vi "Main.vi"() -> ()   [LabVIEW 2020]
doc: "Use this template to build a simple state machine design pattern. Each state executes code and determines which state to transition to."
uses:
  controls/State.ctl
  controls/Data.ctl
  <vilib>/Utility/file.llb/Write Delimited Spreadsheet (string).vi
panel:
  in  "Operator":string(combo)
  in  "Run Lift-Off Pulses":bool
  out "Number of layers":i32
  out "Build":string
  in  "Refresh Supplies":bool
  out "Current now [A]":dbl format="%#.2f"
  in  "Wafer Box":string(combo)="(i)(1)"
  out "Elapsed Time [s]":dbl min=0.0 step=1.0 format="%#.1f"
  in  "Run Lift-Off Pulses\nAfter Etching":bool=TRUE
  in  "Edit Lift-Off Pulses":bool
  in  "Start Etching":bool
  in  "Everyting Correct":bool
  in  "Total Etch Time [s]":u32=2400 step=1
  in  "Wait Time [ms]":u32=2 step=1
  in  "Pulse 2 Time [ms]":u32=2 step=1
  in  "Pulse 1 Time [ms]":u32=2 step=1
  out "[A]":dbl=50.0 min=0.0 max=500.0 step=0.1 format="%#.2g"
  in  "Pulse 2 [mA/cm²]":dbl=50.0 min=0.0 max=900.0 step=0.1 format="%#.3g"
  out "[A]":dbl=50.0 min=0.0 max=500.0 step=0.1 format="%#.2g"
  in  "Pulse 1 [mA/cm²]":dbl=50.0 min=0.0 max=900.0 step=0.1 format="%#.3g"
  out "XY Graph":cluster{"X":dbl[], "Y":dbl[]}[](graph)
  in  "Etch type":T1(tab)
  in  "Current density (mA/cm²)":dbl=30.0 format="%#.2g"
  in  "Current density 1 [mA/cm²]":dbl=50.0 min=0.0 max=500.0 step=0.1 format="%#.2g"
  in  "Current density 2 [mA/cm²]":dbl=200.0 min=0.0 max=500.0 step=0.1 format="%#.2g"
  in  "Pulse time 1 [ms]":u32=2200 step=1
  in  "Pulse time 2 [ms]":u32=350 step=1
  in  "Stop time [ms]":u32=1000 step=1
  in  "Start Current Time [ms]":u32=2000 step=1
  in  "Start Current density [mA/cm²]":dbl=30.0 min=0.0 max=500.0 step=0.1 format="%#.2g"
  in  "Power order":dbl=1.0 min=0.0 step=0.1 format="%#.1g"
  in  "Increment time span [ms]":u32=250 step=1
  in  "Current Density Increment [mA/cm²/s^(power order)]":dbl=1.0 min=0.0 max=500.0 step=0.1 format="%#.6g"
  in  "Etch Surface Area [cm²]":dbl min=0.0 max=1000.0 step=0.1 format="%#.2f"
  in  "Etch Cell":i32(slide) scale=0.0..3.0
  in  "Power Supply":u16(ring)
  in  "Exit":bool
  # "University of Eastern Finland\nJoakim Riikonen / Konstantin Tamarov"
  # "The Ultimate PSi Etching Software"
  # "Etch Cell and Etch Surface Area"
  # "Etch Program"
  # "Lift-Off Pulses"
  # "Start Etching"
  # "Start with short period of contant current to initiate pores"
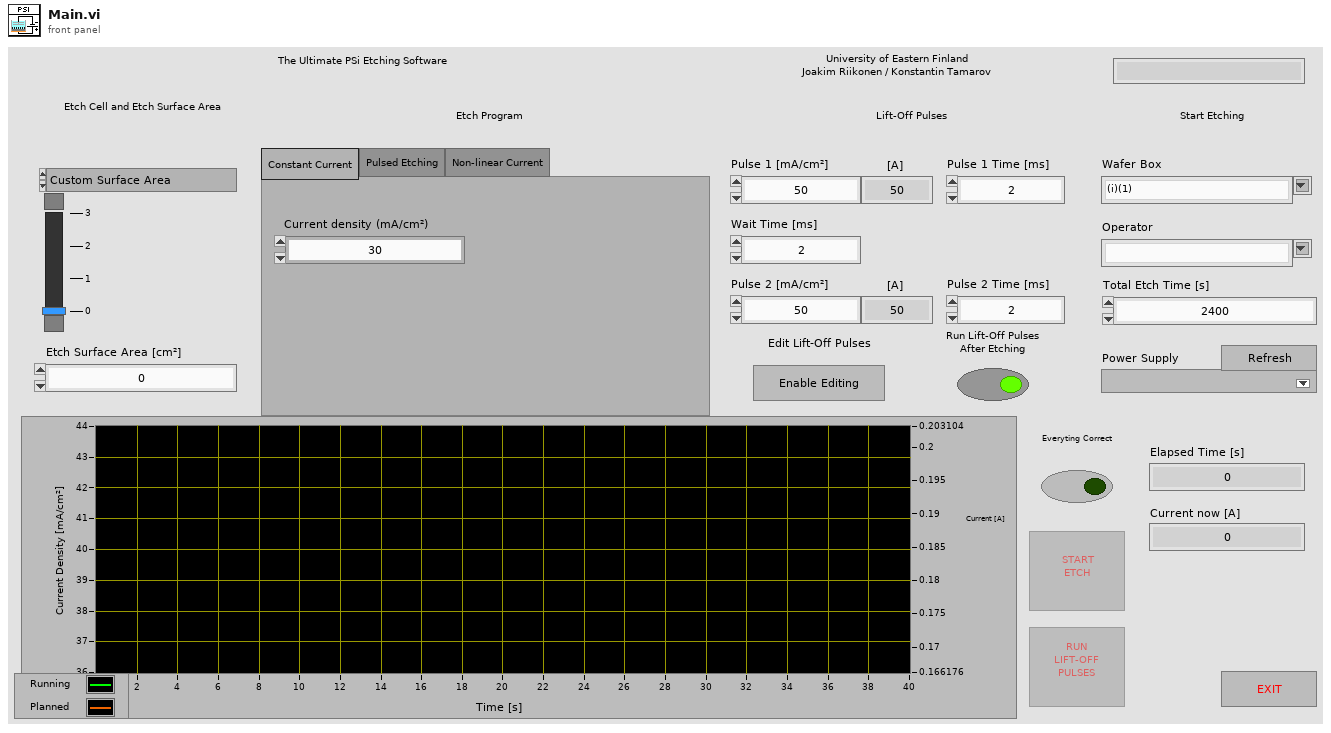
[diagram p1: front panel]
types:
  T1 = enum32{"Constant Current", "Pulsed Etching", "Non-linear Current"}
  T2 = typedef "State.ctl" = enum16{"Initialize", "Wait for Message", "Etch Cell Changed", "LiftOff Pulse Changed", "Enable Editing Pulses Clicked", "Etch Type Changed", "Refresh Supplies Clicked", "Etch Parameters Changed", "Prepare Etch Program", "Check Power Supplies", "Check Max Current", "Prepare Graph", "Before Etch", "Prepare Log", "Etch Running", "Stop Etch Clicked", "LiftOff Pulses", "After Etch", "Exit"}
  T3 = typedef "Data.ctl" = cluster{"Power Supplies":cluster{"Full Name":string[], "Supply Model":string[], "Supply Address":string[], "Max Voltage (V)":dbl[], "Max Current (A)":dbl[]}, "Etch Cell Data":cluster{"Cell Type":string[], "Power Supply Model":string[], "Etch Surface Area (cm2)":dbl[], "LiftOff Pulse 1 (mA/cm2)":dbl[], "LiftOff Time 1 (ms)":u32[], "LiftOff Wait Time 1 (ms)":u32[], "LiftOff Pulse 2 (mA/cm2)":dbl[], "LiftOff Time 2 (ms)":i32[]}, "Etch Program":cluster{"Current Time [ms]":u32[], "Current Density [mA/cm2]":dbl[], "Current [A]":dbl[]}, "Graph Data":cluster{"X":dbl[], "Y":dbl[]}, "Selected VISA":string, "Selected Voltage Limit":dbl, "Log":string[], "Etch Result":string, "Etch Finished Correctly":bool, "Only LiftOff Pulses":bool}
  T4 = enum8{"Enabled", "Disabled", "Disabled and Grayed Out"}
  T5 = cluster{"Current Density [mA/cm2]":dbl[], "Current [A]":dbl[], "Current Time [ms]":u32[]}
  T6 = cluster{"array":string[], "array":string[], "array":string[], "array":dbl[], "array":dbl[]}
  T7 = cluster{"array":string[], "array":string[], "array":dbl[], "array":dbl[], "array":u32[], "array":u32[], "array":dbl[], "array":i32[]}
  T8 = cluster{"array":i32[], "array":dbl[], "array":dbl[]}
  T9 = cluster{"Current Time [ms]":u32[], "Current Density [mA/cm2]":dbl[], "Current [A]":dbl[]}
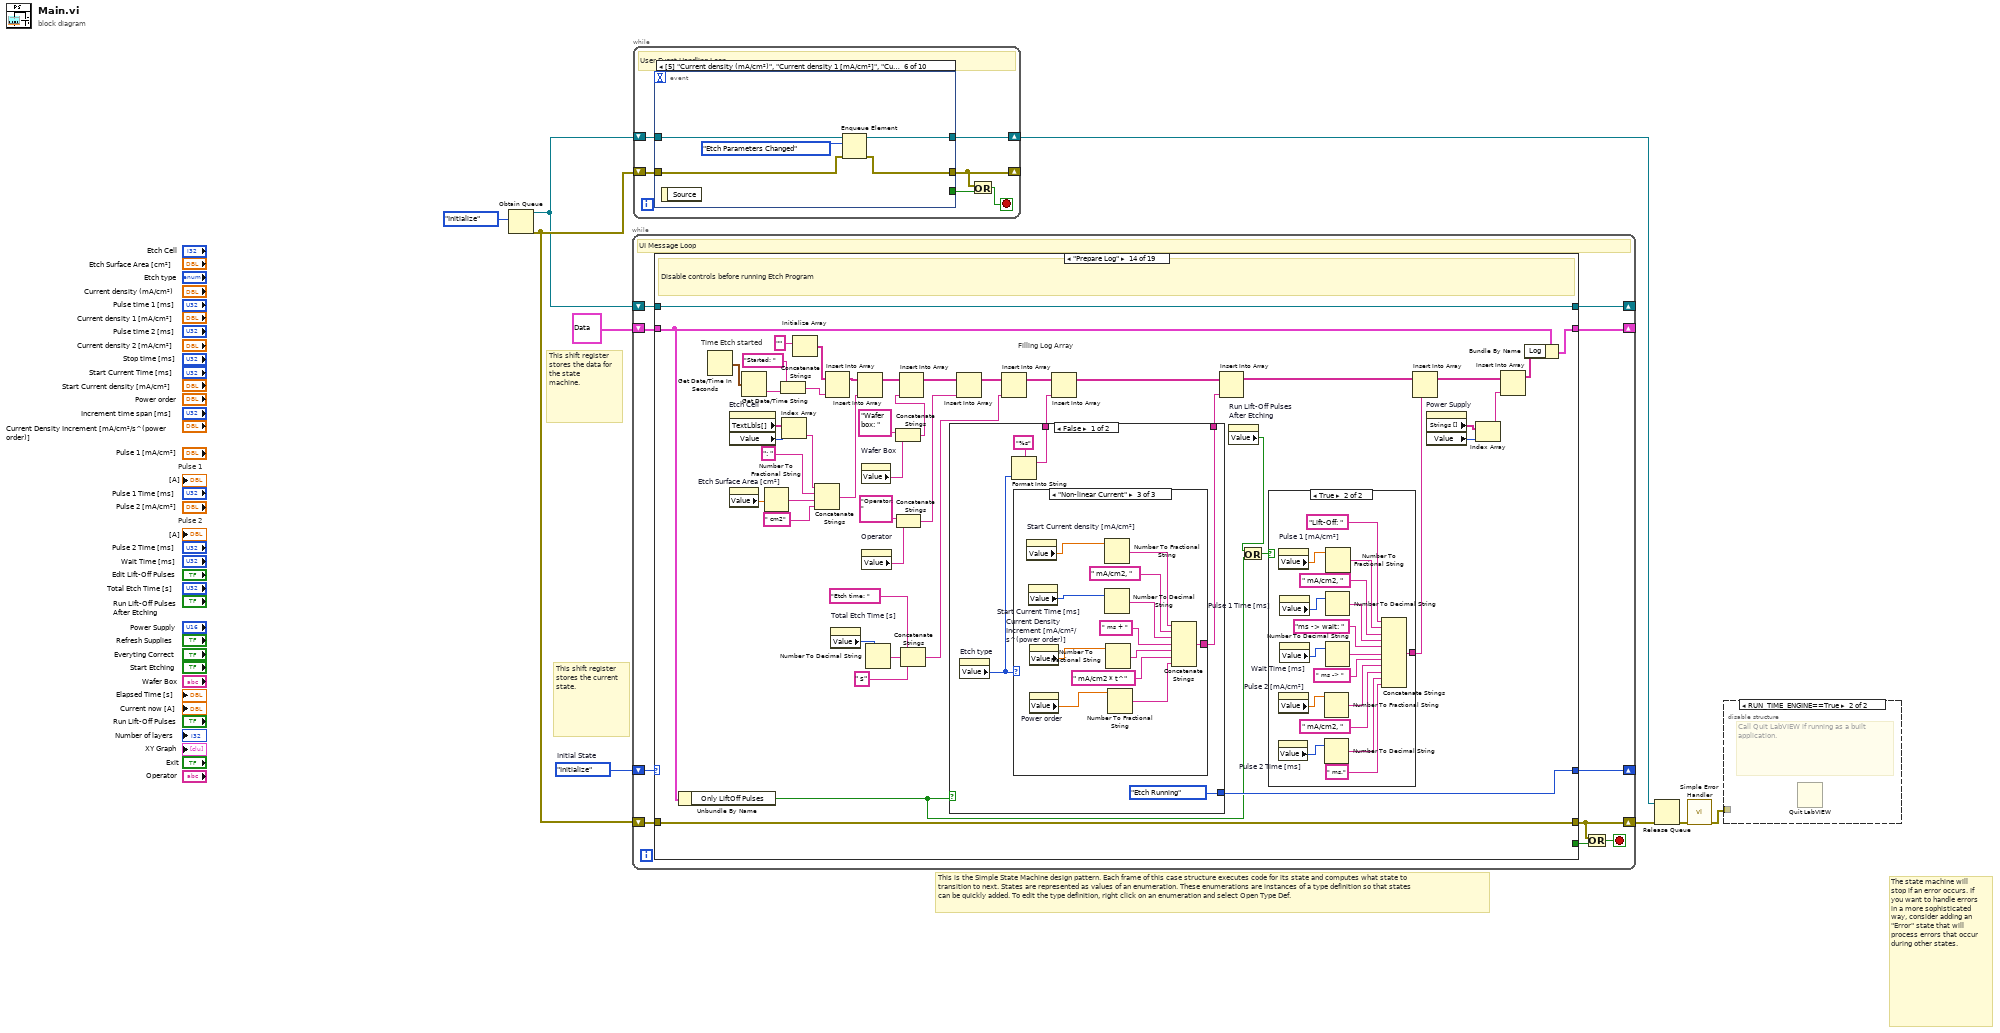
[diagram p0: block diagram]
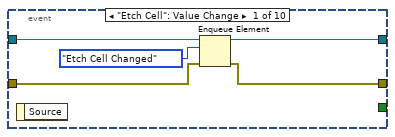
[diagram p2: hidden frame]
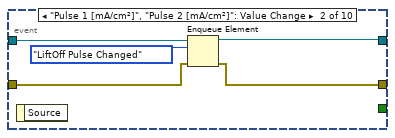
[diagram p3: hidden frame]
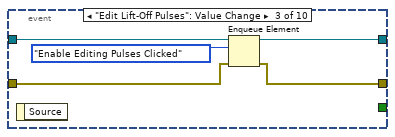
[diagram p4: hidden frame]
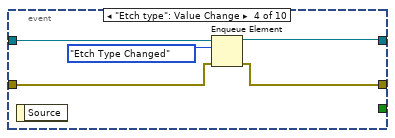
[diagram p5: hidden frame]
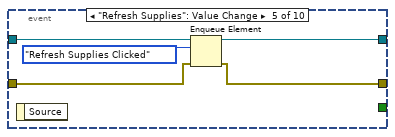
[diagram p6: hidden frame]
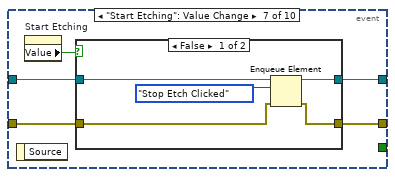
[diagram p7: hidden frame]
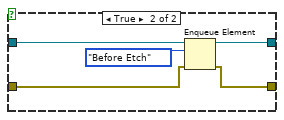
[diagram p8: hidden frame]
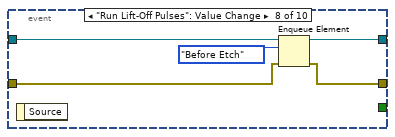
[diagram p9: hidden frame]
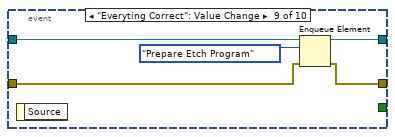
[diagram p10: hidden frame]
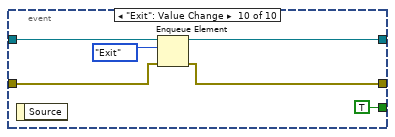
[diagram p11: hidden frame]
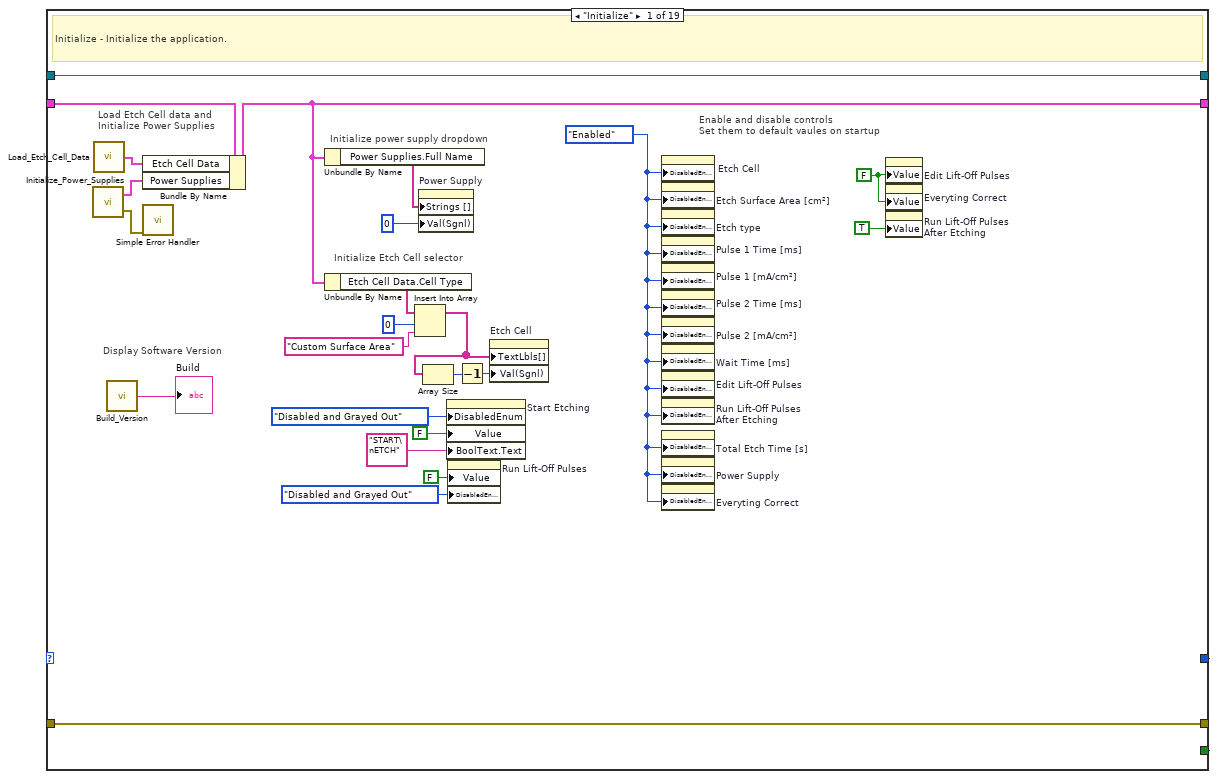
[diagram p13: hidden frame]
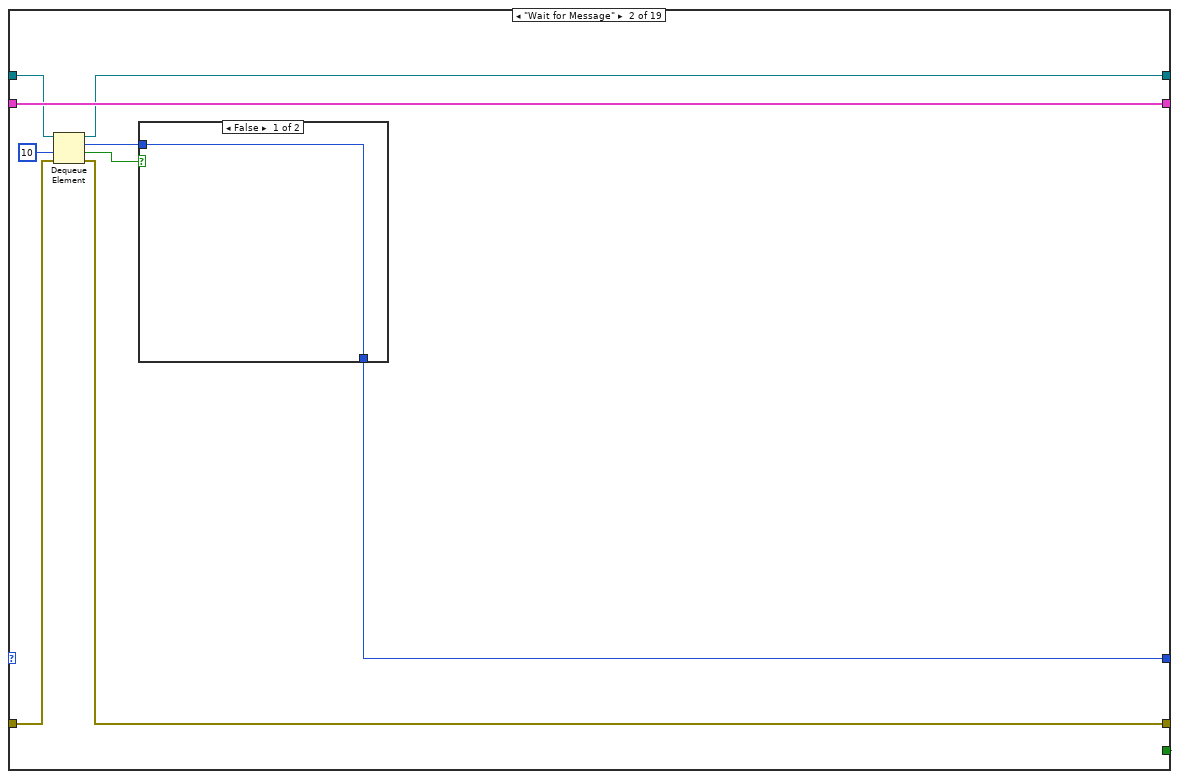
[diagram p14: hidden frame]
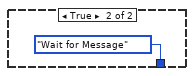
[diagram p15: hidden frame]
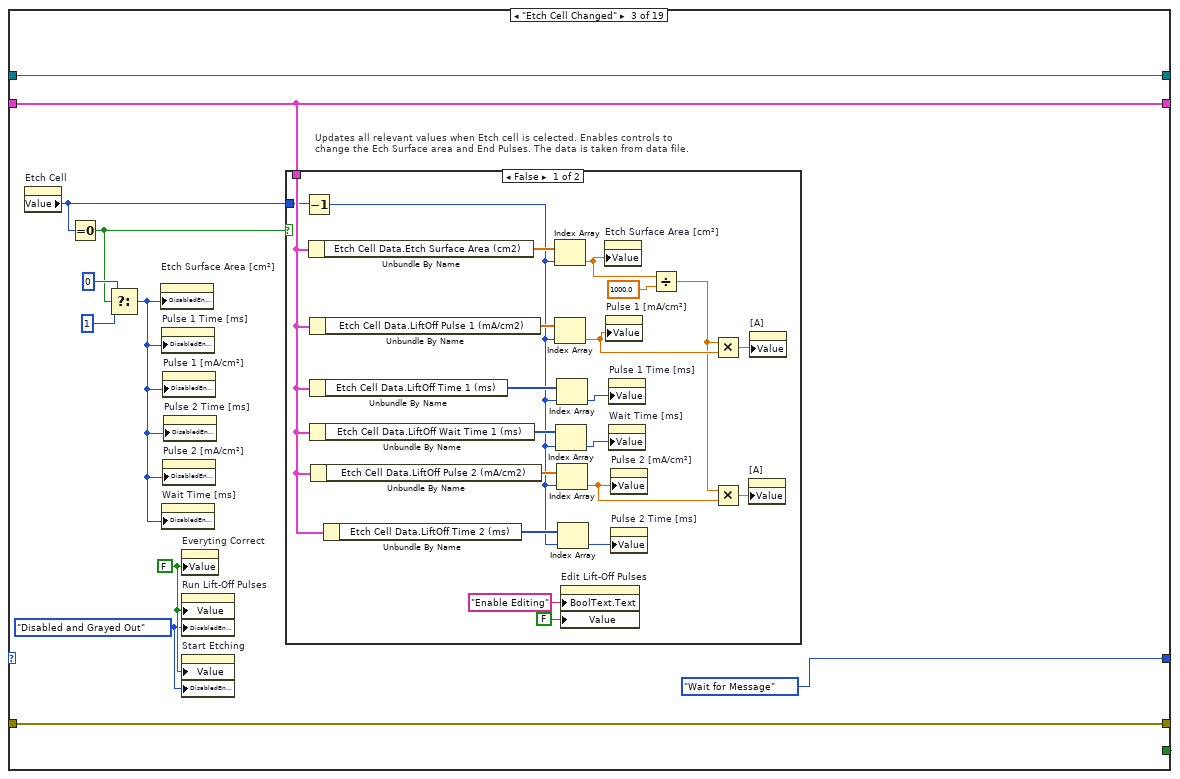
[diagram p16: hidden frame]
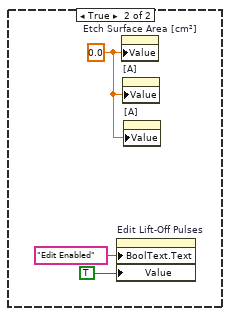
[diagram p17: hidden frame]
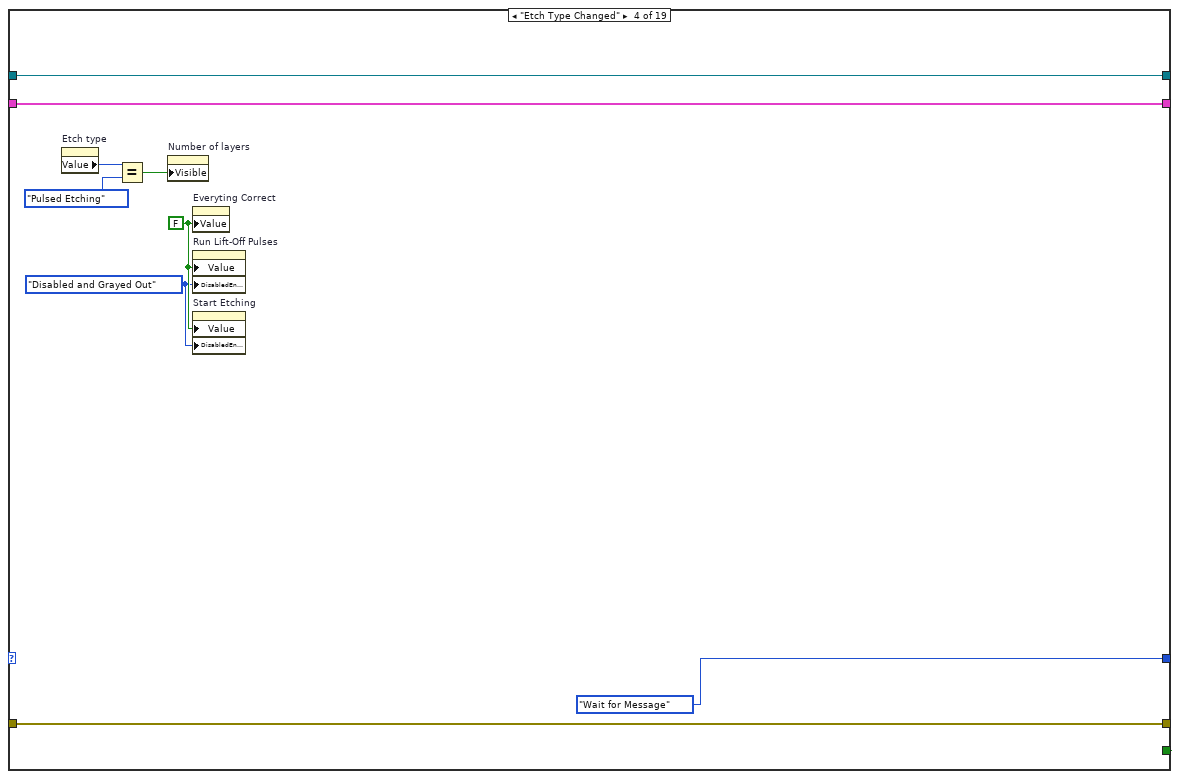
[diagram p18: hidden frame]
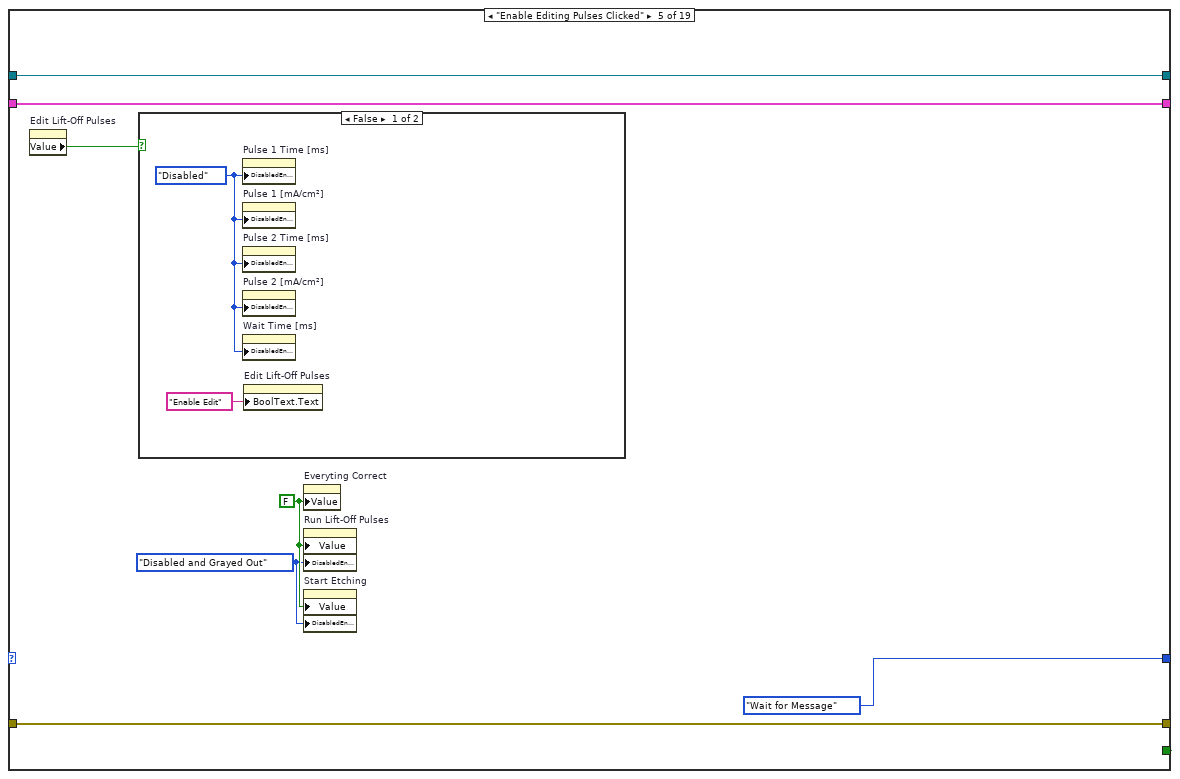
[diagram p19: hidden frame]
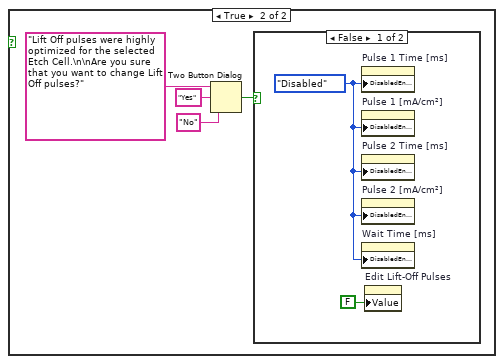
[diagram p20: hidden frame]
diagram:
  w5 = State."Initialize"  # Initial State
  # "Pulse 2"
  # "Pulse 1"
  # "The state machine will stop if an error occurs. If you want to handle errors in a more sophisticated way, consider adding an \"Error\" state that will process errors that occur during other states."
  # "This shift register stores the data for the state machine."
  # "This is the Simple State Machine design pattern. Each frame of this case structure executes code for its state and computes what state to transition to next. States are represented as values of an enumeration. These enumerations are instances of a type definition so that states can be quickly added. To edit the type definition, right click on an enumeration and select Open Type Def."
  # "This shift register stores the current state."
  n1 = Obtain Queue(element data type=State."Initialize" ("element")) -> (queue out=w3:refnum<queue>, error out=w7:errorcluster)  [unwired: 4 in, 1 out]
  n2 = while {
    shift-right: [w19] -> _
    shift-left: w5 -> [w12]
    shift-right: [w13] -> _
    shift-left: T3 {"Power Supplies"={"Full Name"=[], "Supply Model"=[], "Supply Address"=[], "Max Voltage (V)"=[], "Max Current (A)"=[]}, "Etch Cell Data"={"Cell Type"=[], "Power Supply Model"=[], "Etch Surface Area (cm2)"=[], "LiftOff Pulse 1 (mA/cm2)"=[], "LiftOff Time 1 (ms)"=[], "LiftOff Wait Time 1 (ms)"=[], "LiftOff Pulse 2 (mA/cm2)"=[], "LiftOff Time 2 (ms)"=[]}, "Etch Program"={"Current Time [ms]"=[], "Current Density [mA/cm2]"=[], "Current [A]"=[]}, "Graph Data"={"X"=[], "Y"=[]}, "Selected VISA"="", "Selected Voltage Limit"=0.0, "Log"=[], "Etch Result"="", "Etch Finished Correctly"=FALSE, "Only LiftOff Pulses"=FALSE} ("Data") -> [w14]
    shift-right: [w15] -> w2
    shift-left: w7 -> [w18]
    shift-right: [w10] -> _
    shift-left: w3 -> [w11]
    stop <- w16 stop-if-true
    # "UI Message Loop"
    n3 = case shown="\"Prepare Log\"" w12 {
      tunnel: [w45 w46 State."Wait for Message" ("(Value Not Used)") State."Wait for Message" ("(Value Not Used)") State."Wait for Message" ("(Value Not Used)") State."Wait for Message" ("(Value Not Used)") State."Wait for Message" ("(Value Not Used)") State."Wait for Message" ("(Value Not Used)") w156 w288 w325 w384 State."Prepare Log" ("Next State") w437 w591 State."After Etch" ("next state") w703 w746 State."LiftOff Pulses" ("(Value Not Used)")] -> w19
      tunnel: [w44 FALSE ("Stop Loop?") FALSE ("Stop Loop?") FALSE ("Stop Loop?") FALSE ("Stop Loop?") FALSE ("Stop Loop?") FALSE ("Stop Loop?") FALSE ("Stop Loop?") w161 FALSE ("Stop Loop?") FALSE ("Stop Loop?") FALSE ("Stop Loop?") w424 w439 w590 FALSE ("Stop Loop?") w706 w744 FALSE ("Stop Loop?")] -> w17
      tunnel: w14 -> [w43 w55 w63 w103 w111 w135 w141 w154 w158 w292 w328 w365 w413 w438 w557 w648 w705 w745 w751]
      tunnel: [w24 w55 w63 w103 w111 w135 w140 w154 w157 w292 w328 w364 w416 w458 w576 w648 w705 w745 w751] -> w13
      tunnel: w18 -> [w26 w52 w69 w102 w110 w134 w137 w153 w160 w296 w331 w391 w422 w443 w538 w653 w707 w743 w750]
      tunnel: [w26 w51 w69 w102 w110 w134 w137 w153 w160 w296 w331 w391 w422 w443 w537 w653 w707 w743 w750] -> w15
      tunnel: w11 -> [w22 w54 w62 w97 w109 w133 w147 w152 w155 w287 w314 w346 w420 w440 w545 w647 w704 w742 w749]
      tunnel: [w22 w53 w62 w97 w109 w133 w147 w152 w155 w287 w314 w346 w420 w440 w544 w647 w704 w742 w749] -> w10
      frame "Initialize" {
        w31 = T4."Enabled" ("Disabled")
        w37 = FALSE ("Edit Lift-Off Pulses")
        w44 = FALSE  # Stop Loop?
        w45 = State."Wait for Message"  # Next State
        # "Initialize Etch Cell selector"
        # "Enable and disable controls\nSet them to default vaules on startup"
        # "Initialize power supply dropdown"
        # "Display Software Version"
        # "Load Etch Cell data and\nInitialize Power Supplies"
        # "Initialize - Initialize the application."
        n4 = call "Initialize_Power_Supplies.vi"() -> ("error out"=w20:errorcluster, "Available Power Supplies"=w21:T6)  [unwired: 2 in]
        n5 = call "Load_Etch_Cell_Data.vi"() -> ("Etch Cell Data"=w38:T7)  [unwired: 1 in]
        n6 = call "Build_Version.vi"() -> ("Version"=→"Build":string)  [unwired: 1 in]
        n7 = Bundle By Name(cluster=w43, "Etch Cell Data"=w38, "Power Supplies"=w21) -> (w24:T3)
        n8 = call <vilib>:"Simple Error Handler.vi"("error in (no error)"=w20) -> ()  [unwired: 4 in, 5 out]
        n9 = Unbundle By Name(w24) -> ("Power Supplies.Full Name"=w25:string[])
        n10 = Unbundle By Name(w24) -> ("Etch Cell Data.Cell Type"=w42:string[])
        n11 = Insert Into Array(array=w42, index=0, new element="Custom Surface Area" ("new element/subarray")) -> (w39:string[])
        n12 = property on="Power Supply" class="Ring (strict)"("Strings []"=w25, "Val(Sgnl)"=u16 0 ("Value (Signaling)")) -> ()  [unwired: 2 in, 2 out]
        n13 = Array Size(array=w39) -> (size(s)=w33:i32)
        n14 = property on="Start Etching" class="Bool (strict)"("DisabledEnum"=T4."Disabled and Grayed Out" ("Disabled"), "Value"=FALSE ("Start Etching"), "BoolText.Text"="START\nETCH" ("Boolean Text.Text")) -> ()  [unwired: 2 in, 2 out]
        n15 = property on="Run Lift-Off Pulses" class="Bool (strict)"("Value"=FALSE ("Run Lift-Off Pulses"), "DisabledEnum"=T4."Disabled and Grayed Out" ("Disabled")) -> ()  [unwired: 2 in, 2 out]
        n16 = Decrement(x=w33) -> (x-1=w23:i32)
        n17 = property on="Etch Cell" class="Slide (strict)"("TextLbls[]"=w39, "Val(Sgnl)"=w23) -> ()  [unwired: 2 in, 2 out]
        n18 = property on="Etch Cell" class="Slide (strict)"("DisabledEnum"=w31) -> ()  [unwired: 2 in, 2 out]
        n19 = property on="Etch Surface Area [cm²]" class="DigNum (strict)"("DisabledEnum"=w31) -> ()  [unwired: 2 in, 2 out]
        n20 = property on="Etch type" class="TabCtl (strict)"("DisabledEnum"=w31) -> ()  [unwired: 2 in, 2 out]
        n21 = property on="Pulse 1 Time [ms]" class="DigNum (strict)"("DisabledEnum"=w31) -> ()  [unwired: 2 in, 2 out]
        n22 = property on="Pulse 1 [mA/cm²]" class="DigNum (strict)"("DisabledEnum"=w31) -> ()  [unwired: 2 in, 2 out]
        n23 = property on="Pulse 2 Time [ms]" class="DigNum (strict)"("DisabledEnum"=w31) -> ()  [unwired: 2 in, 2 out]
        n24 = property on="Pulse 2 [mA/cm²]" class="DigNum (strict)"("DisabledEnum"=w31) -> ()  [unwired: 2 in, 2 out]
        n25 = property on="Wait Time [ms]" class="DigNum (strict)"("DisabledEnum"=w31) -> ()  [unwired: 2 in, 2 out]
        n26 = property on="Edit Lift-Off Pulses" class="Bool (strict)"("DisabledEnum"=w31) -> ()  [unwired: 2 in, 2 out]
        n27 = property on="Run Lift-Off Pulses\nAfter Etching" class="Bool (strict)"("DisabledEnum"=w31) -> ()  [unwired: 2 in, 2 out]
        n28 = property on="Total Etch Time [s]" class="DigNum (strict)"("DisabledEnum"=w31) -> ()  [unwired: 2 in, 2 out]
        n29 = property on="Power Supply" class="Ring (strict)"("DisabledEnum"=w31) -> ()  [unwired: 2 in, 2 out]
        n30 = property on="Everyting Correct" class="Bool (strict)"("DisabledEnum"=w31) -> ()  [unwired: 2 in, 2 out]
        n31 = property on="Edit Lift-Off Pulses" class="Bool (strict)"("Value"=w37) -> ()  [unwired: 2 in, 2 out]
        n32 = property on="Everyting Correct" class="Bool (strict)"("Value"=w37) -> ()  [unwired: 2 in, 2 out]
        n33 = property on="Run Lift-Off Pulses\nAfter Etching" class="Bool (strict)"("Value"=TRUE ("Run Lift-Off Pulses\nAfter Etching")) -> ()  [unwired: 2 in, 2 out]
      }
      frame "Wait for Message" {
        n34 = Dequeue Element(queue=w54, timeout in ms (-1)=10, error in (no error)=w52) -> (queue out=w53:refnum<queue>, element=w47:T2, timed out?=w48:bool, error out=w51:errorcluster)
        n35 = case shown="False" w48 {
          tunnel: w47 -> [w56 _]
          tunnel: [w56 State."Wait for Message" ("(Value Not Used)")] -> w46
          frame False {
          }
          frame True {
          }
        }
      }
      frame "Etch Cell Changed" {
        w58 = T4."Disabled and Grayed Out" ("Disabled")
        w59 = FALSE ("Everyting Correct")
        # "Updates all relevant values when Etch cell is celected. Enables controls to\nchange the Ech Surface area and End Pulses. The data is taken from data file."
        n36 = property on="Etch Cell" class="Slide (strict)"() -> ("Value"=w64:i32)  [unwired: 2 in, 2 out]
        n37 = Equal To 0?(x=w64) -> (x = 0?=w65:bool)
        n38 = Select(t=i8 0, s=w65, f=i8 1) -> (s? t:f=w68:i8)
        n39 = property on="Etch Surface Area [cm²]" class="DigNum (strict)"("DisabledEnum"=w68) -> ()  [unwired: 2 in, 2 out]
        n40 = property on="Pulse 1 Time [ms]" class="DigNum (strict)"("DisabledEnum"=w68) -> ()  [unwired: 2 in, 2 out]
        n41 = property on="Wait Time [ms]" class="DigNum (strict)"("DisabledEnum"=w68) -> ()  [unwired: 2 in, 2 out]
        n42 = property on="Pulse 1 [mA/cm²]" class="DigNum (strict)"("DisabledEnum"=w68) -> ()  [unwired: 2 in, 2 out]
        n43 = property on="Pulse 2 [mA/cm²]" class="DigNum (strict)"("DisabledEnum"=w68) -> ()  [unwired: 2 in, 2 out]
        n44 = property on="Pulse 2 Time [ms]" class="DigNum (strict)"("DisabledEnum"=w68) -> ()  [unwired: 2 in, 2 out]
        n45 = property on="Everyting Correct" class="Bool (strict)"("Value"=w59) -> ()  [unwired: 2 in, 2 out]
        n46 = property on="Run Lift-Off Pulses" class="Bool (strict)"("Value"=w59, "DisabledEnum"=w58) -> ()  [unwired: 2 in, 2 out]
        n47 = property on="Start Etching" class="Bool (strict)"("Value"=w59, "DisabledEnum"=w58) -> ()  [unwired: 2 in, 2 out]
        n48 = case shown="False" w65 {
          tunnel: w64 -> [w73 _]
          tunnel: w63 -> [w86 _]
          frame False {
            n49 = Decrement(x=w73) -> (x-1=w72:i32)
            n50 = Unbundle By Name(w86) -> ("Etch Cell Data.Etch Surface Area (cm2)"=w90:dbl[])
            n51 = Unbundle By Name(w86) -> ("Etch Cell Data.LiftOff Pulse 1 (mA/cm2)"=w89:dbl[])
            n52 = Unbundle By Name(w86) -> ("Etch Cell Data.LiftOff Time 1 (ms)"=w88:u32[])
            n53 = Unbundle By Name(w86) -> ("Etch Cell Data.LiftOff Wait Time 1 (ms)"=w85:u32[])
            n54 = Unbundle By Name(w86) -> ("Etch Cell Data.LiftOff Pulse 2 (mA/cm2)"=w84:dbl[])
            n55 = Unbundle By Name(w86) -> ("Etch Cell Data.LiftOff Time 2 (ms)"=w83:i32[])
            n56 = Index Array(array=w90, index=w72) -> (element=w78:dbl)
            n57 = Index Array(array=w89, index=w72) -> (element=w80:dbl)
            n58 = Index Array(array=w85, index=w72) -> (element=w82:u32)
            n59 = Index Array(array=w88, index=w72) -> (element=w87:u32)
            n60 = Index Array(array=w84, index=w72) -> (element=w79:dbl)
            n61 = Index Array(array=w83, index=w72) -> (element=w81:i32)
            n62 = property on="Edit Lift-Off Pulses" class="Bool (strict)"("BoolText.Text"="Enable Editing" ("Boolean Text.Text"), "Value"=FALSE ("Edit Lift-Off Pulses")) -> ()  [unwired: 2 in, 2 out]
            n63 = property on="Etch Surface Area [cm²]" class="DigNum (strict)"("Value"=w78) -> ()  [unwired: 2 in, 2 out]
            n64 = property on="Pulse 1 [mA/cm²]" class="DigNum (strict)"("Value"=w80) -> ()  [unwired: 2 in, 2 out]
            n65 = property on="Pulse 1 Time [ms]" class="DigNum (strict)"("Value"=w87) -> ()  [unwired: 2 in, 2 out]
            n66 = property on="Wait Time [ms]" class="DigNum (strict)"("Value"=w82) -> ()  [unwired: 2 in, 2 out]
            n67 = property on="Pulse 2 [mA/cm²]" class="DigNum (strict)"("Value"=w79) -> ()  [unwired: 2 in, 2 out]
            n68 = property on="Pulse 2 Time [ms]" class="DigNum (strict)"("Value"=w81) -> ()  [unwired: 2 in, 2 out]
            n69 = Divide(x=w78, y=1000.0) -> (x/y=w77:dbl)
            n70 = Multiply(x=w77, y=w80) -> (x*y=w71:dbl)
            n71 = Multiply(x=w77, y=w79) -> (x*y=w70:dbl)
            n72 = property on="[A]" class="DigNum (strict)"("Value"=w70) -> ()  [unwired: 2 in, 2 out]
            n73 = property on="[A]" class="DigNum (strict)"("Value"=w71) -> ()  [unwired: 2 in, 2 out]
          }
          frame True {
            w91 = 0.0 ("Etch Surface Area (cm²)")
            n74 = property on="Edit Lift-Off Pulses" class="Bool (strict)"("BoolText.Text"="Edit Enabled" ("Boolean Text.Text"), "Value"=TRUE ("Edit Lift-Off Pulses")) -> ()  [unwired: 2 in, 2 out]
            n75 = property on="Etch Surface Area [cm²]" class="DigNum (strict)"("Value"=w91) -> ()  [unwired: 2 in, 2 out]
            n76 = property on="[A]" class="DigNum (strict)"("Value"=w91) -> ()  [unwired: 2 in, 2 out]
            n77 = property on="[A]" class="DigNum (strict)"("Value"=w91) -> ()  [unwired: 2 in, 2 out]
          }
        }
      }
      frame "Etch Type Changed" {
        w100 = T4."Disabled and Grayed Out" ("Disabled")
        w101 = FALSE ("Everyting Correct")
        n78 = property on="Etch type" class="TabCtl (strict)"() -> ("Value"=w96:T1)  [unwired: 2 in, 2 out]
        n79 = Equal?(x=w96, y=T1."Pulsed Etching") -> (x = y?=w94:bool)
        n80 = property on="Number of layers" class="DigNum (strict)"("Visible"=w94) -> ()  [unwired: 2 in, 2 out]
        n81 = property on="Everyting Correct" class="Bool (strict)"("Value"=w101) -> ()  [unwired: 2 in, 2 out]
        n82 = property on="Run Lift-Off Pulses" class="Bool (strict)"("Value"=w101, "DisabledEnum"=w100) -> ()  [unwired: 2 in, 2 out]
        n83 = property on="Start Etching" class="Bool (strict)"("Value"=w101, "DisabledEnum"=w100) -> ()  [unwired: 2 in, 2 out]
      }
      frame "Enable Editing Pulses Clicked" {
        w105 = T4."Disabled and Grayed Out" ("Disabled")
        w106 = FALSE ("Everyting Correct")
        n84 = property on="Edit Lift-Off Pulses" class="Bool (strict)"() -> ("Value"=w104:bool)  [unwired: 2 in, 2 out]
        n85 = case shown="False" w104 {
          frame False {
            w112 = T4."Disabled" ("Disabled")
            n86 = property on="Pulse 1 Time [ms]" class="DigNum (strict)"("DisabledEnum"=w112) -> ()  [unwired: 2 in, 2 out]
            n87 = property on="Pulse 1 [mA/cm²]" class="DigNum (strict)"("DisabledEnum"=w112) -> ()  [unwired: 2 in, 2 out]
            n88 = property on="Pulse 2 Time [ms]" class="DigNum (strict)"("DisabledEnum"=w112) -> ()  [unwired: 2 in, 2 out]
            n89 = property on="Pulse 2 [mA/cm²]" class="DigNum (strict)"("DisabledEnum"=w112) -> ()  [unwired: 2 in, 2 out]
            n90 = property on="Wait Time [ms]" class="DigNum (strict)"("DisabledEnum"=w112) -> ()  [unwired: 2 in, 2 out]
            n91 = property on="Edit Lift-Off Pulses" class="Bool (strict)"("BoolText.Text"="Enable Edit" ("Boolean Text.Text")) -> ()  [unwired: 2 in, 2 out]
          }
          frame True {
            n92 = Two Button Dialog(message="Lift Off pulses were highly optimized for the selected Etch Cell.\n\nAre you sure that you want to change Lift Off pulses?", 1:"No" ("F button name (\"Cancel\")"), 2:"Yes" ("T button name (\"OK\")")) -> (T button?=w117:bool)
            n93 = case shown="False" w117 {
              frame False {
                w119 = T4."Disabled" ("Disabled")
                n94 = property on="Pulse 1 Time [ms]" class="DigNum (strict)"("DisabledEnum"=w119) -> ()  [unwired: 2 in, 2 out]
                n95 = property on="Pulse 1 [mA/cm²]" class="DigNum (strict)"("DisabledEnum"=w119) -> ()  [unwired: 2 in, 2 out]
                n96 = property on="Pulse 2 Time [ms]" class="DigNum (strict)"("DisabledEnum"=w119) -> ()  [unwired: 2 in, 2 out]
                n97 = property on="Pulse 2 [mA/cm²]" class="DigNum (strict)"("DisabledEnum"=w119) -> ()  [unwired: 2 in, 2 out]
                n98 = property on="Wait Time [ms]" class="DigNum (strict)"("DisabledEnum"=w119) -> ()  [unwired: 2 in, 2 out]
                n99 = property on="Edit Lift-Off Pulses" class="Bool (strict)"("Value"=FALSE ("Edit Lift-Off Pulses")) -> ()  [unwired: 2 in, 2 out]
              }
              frame True {
                w121 = T4."Enabled" ("Disabled")
                n100 = property on="Pulse 1 [mA/cm²]" class="DigNum (strict)"("DisabledEnum"=w121) -> ()  [unwired: 2 in, 2 out]
                n101 = property on="Pulse 1 Time [ms]" class="DigNum (strict)"("DisabledEnum"=w121) -> ()  [unwired: 2 in, 2 out]
                n102 = property on="Wait Time [ms]" class="DigNum (strict)"("DisabledEnum"=w121) -> ()  [unwired: 2 in, 2 out]
                n103 = property on="Pulse 2 Time [ms]" class="DigNum (strict)"("DisabledEnum"=w121) -> ()  [unwired: 2 in, 2 out]
                n104 = property on="Pulse 2 [mA/cm²]" class="DigNum (strict)"("DisabledEnum"=w121) -> ()  [unwired: 2 in, 2 out]
                n105 = property on="Edit Lift-Off Pulses" class="Bool (strict)"("BoolText.Text"="Editing Enabled" ("Boolean Text.Text")) -> ()  [unwired: 2 in, 2 out]
              }
            }
          }
        }
        n106 = property on="Everyting Correct" class="Bool (strict)"("Value"=w106) -> ()  [unwired: 2 in, 2 out]
        n107 = property on="Run Lift-Off Pulses" class="Bool (strict)"("Value"=w106, "DisabledEnum"=w105) -> ()  [unwired: 2 in, 2 out]
        n108 = property on="Start Etching" class="Bool (strict)"("Value"=w106, "DisabledEnum"=w105) -> ()  [unwired: 2 in, 2 out]
      }
      frame "LiftOff Pulse Changed" {
        w122 = T4."Disabled and Grayed Out" ("Disabled")
        w123 = FALSE ("Everyting Correct")
        n109 = property on="Etch Surface Area [cm²]" class="DigNum (strict)"() -> ("Value"=w129:dbl)  [unwired: 2 in, 2 out]
        n110 = property on="Pulse 1 [mA/cm²]" class="DigNum (strict)"() -> ("Value"=w131:dbl)  [unwired: 2 in, 2 out]
        n111 = property on="Pulse 2 [mA/cm²]" class="DigNum (strict)"() -> ("Value"=w130:dbl)  [unwired: 2 in, 2 out]
        n112 = Divide(x=w129, y=1000.0) -> (x/y=w128:dbl)
        n113 = Multiply(x=w128, y=w131) -> (x*y=w126:dbl)
        n114 = Multiply(x=w128, y=w130) -> (x*y=w125:dbl)
        n115 = property on="[A]" class="DigNum (strict)"("Value"=w126) -> ()  [unwired: 2 in, 2 out]
        n116 = property on="[A]" class="DigNum (strict)"("Value"=w125) -> ()  [unwired: 2 in, 2 out]
        n117 = property on="Everyting Correct" class="Bool (strict)"("Value"=w123) -> ()  [unwired: 2 in, 2 out]
        n118 = property on="Run Lift-Off Pulses" class="Bool (strict)"("Value"=w123, "DisabledEnum"=w122) -> ()  [unwired: 2 in, 2 out]
        n119 = property on="Start Etching" class="Bool (strict)"("Value"=w123, "DisabledEnum"=w122) -> ()  [unwired: 2 in, 2 out]
      }
      frame "Refresh Supplies Clicked" {
        w142 = T4."Disabled and Grayed Out" ("Disabled")
        w143 = FALSE ("Everyting Correct")
        # "Initialize power supply dropdown"
        n120 = call "Initialize_Power_Supplies.vi"() -> ("error out"=w136:errorcluster, "Available Power Supplies"=w139:T6)  [unwired: 2 in]
        n121 = Bundle By Name(cluster=w141, "Power Supplies"=w139) -> (w140:T3)
        n122 = call <vilib>:"General Error Handler.vi"("error in (no error)"=w136) -> ()  [unwired: 10 in, 5 out]
        n123 = Unbundle By Name(w140) -> ("Power Supplies.Full Name"=w144:string[])
        n124 = property on="Power Supply" class="Ring (strict)"("Strings []"=w144, "Val(Sgnl)"=u16 0 ("Value (Signaling)")) -> ()  [unwired: 2 in, 2 out]
        n125 = property on="Everyting Correct" class="Bool (strict)"("Value"=w143) -> ()  [unwired: 2 in, 2 out]
        n126 = property on="Run Lift-Off Pulses" class="Bool (strict)"("Value"=w143, "DisabledEnum"=w142) -> ()  [unwired: 2 in, 2 out]
        n127 = property on="Start Etching" class="Bool (strict)"("Value"=w143, "DisabledEnum"=w142) -> ()  [unwired: 2 in, 2 out]
      }
      frame "Etch Parameters Changed" {
        w148 = T4."Disabled and Grayed Out" ("Disabled")
        w149 = FALSE ("Everyting Correct")
        n128 = property on="Everyting Correct" class="Bool (strict)"("Value"=w149) -> ()  [unwired: 2 in, 2 out]
        n129 = property on="Run Lift-Off Pulses" class="Bool (strict)"("Value"=w149, "DisabledEnum"=w148) -> ()  [unwired: 2 in, 2 out]
        n130 = property on="Start Etching" class="Bool (strict)"("Value"=w149, "DisabledEnum"=w148) -> ()  [unwired: 2 in, 2 out]
      }
      frame "Prepare Etch Program" {
        w161 = FALSE  # Stop Loop?
        # "Checks user entered data is correct and builds up etch program."
        n131 = property on="Everyting Correct" class="Bool (strict)"() -> ("Value"=w159:bool)  [unwired: 2 in, 2 out]
        n132 = case shown="True" w159 {
          tunnel: w158 -> [w170 w173]
          tunnel: [w169 w172] -> w157
          tunnel: [w167 w171] -> w156
          frame False {
            w163 = T4."Disabled and Grayed Out" ("Disabled")
            w167 = State."Wait for Message"  # Next State
            # "Go to After Etch state to\nenable possibly disabled \ncontrols"
            n133 = property on="Start Etching" class="Bool (strict)"("Value"=FALSE ("Start Etching"), "BoolText.Text"="START\nETCH" ("Boolean Text.Text"), "DisabledEnum"=w163) -> ()  [unwired: 2 in, 2 out]
            n134 = property on="Run Lift-Off Pulses" class="Bool (strict)"("Value"=FALSE ("Run Lift-Off Pulses"), "DisabledEnum"=w163, "BoolText.Text"="RUN\nLIFT-OFF\nPULSES" ("Boolean Text.Text")) -> ()  [unwired: 2 in, 2 out]
            n135 = Bundle By Name(cluster=w170, "Etch Program"=T5 {"Current Density [mA/cm2]"=[], "Current [A]"=[], "Current Time [ms]"=[]}) -> (w169:T3)
          }
          frame True {
            w171 = State."Check Max Current"  # Next State
            # "Build up etch program"
            n136 = property on="Etch type" class="TabCtl (strict)"() -> ("Value"=w174:T1)  [unwired: 2 in, 2 out]
            n137 = case shown="\"Constant Current\", Default" w174 {
              tunnel: w173 -> [w186 w205 w261]
              tunnel: [w185 w204 w260] -> w172
              frame "Constant Current", Default {
                w183 = 100 ("y")
                # "100 ms time step"
                n138 = property on="Total Etch Time [s]" class="DigNum (strict)"() -> ("Value"=w189:u32)  [unwired: 2 in, 2 out]
                n139 = property on="Current density (mA/cm²)" class="DigNum (strict)"() -> ("Value"=w180:dbl)  [unwired: 2 in, 2 out]
                n140 = property on="Etch Surface Area [cm²]" class="DigNum (strict)"() -> ("Value"=w190:dbl)  [unwired: 2 in, 2 out]
                n141 = Multiply(x=w189, y=1000) -> (x*y=w184:u32)
                n142 = Multiply(x=w180, y=w190) -> (x*y=w192:dbl)
                n143 = Divide(x=w184, y=w183) -> (x/y=w182:dbl)
                n144 = Divide(x=w192, y=1000.0) -> (x/y=w179:dbl)
                n145 = Round To Nearest(number=w182) -> (nearest integer value=w181:dbl)
                n146 = To Long Integer(number=w181) -> (32bit integer=w178:i32)
                n147 = Initialize Array(w183, w178) -> (w177:i32[])
                n148 = Initialize Array(w180, w178) -> (w176:dbl[])
                n149 = Initialize Array(w179, w178) -> (w175:dbl[])
                n150 = Bundle(w177, w176, w175) -> (w187:cluster{i32[], dbl[], dbl[]})  [unwired: 1 in]
                n151 = Bundle By Name(cluster=w186, "Etch Program"=w187) -> (w185:T3)
              }
              frame "Pulsed Etching" {
                # "Array for \ncurrents"
                # "Array for \ncurrent densities"
                # "Array for pulse \nand stop times"
                n152 = property on="Total Etch Time [s]" class="DigNum (strict)"() -> ("Value"=w203:u32)  [unwired: 2 in, 2 out]
                n153 = Multiply(x=w203, y=1000) -> (x*y=w201:u32)
                n154 = while {
                  tunnel: w201 -> [w236]
                  shift-right: [w232] -> _
                  shift-left: u32 0 -> [w233]
                  shift-right: [w225] -> w196
                  shift-left: i32[] [] ("array") -> [w231]
                  shift-right: [w213] -> w194
                  shift-left: dbl[] [] ("array") -> [w218]
                  shift-right: [w206] -> w195
                  shift-left: dbl[] [] ("array") -> [w207]
                  stop <- w235 stop-if-true
                  n155 = property on="Etch Surface Area [cm²]" class="DigNum (strict)"() -> ("Value"=w224:dbl)  [unwired: 2 in, 2 out]
                  n156 = property on="Pulse time 1 [ms]" class="DigNum (strict)"() -> ("Value"=w230:u32)  [unwired: 2 in, 2 out]
                  n157 = property on="Pulse time 2 [ms]" class="DigNum (strict)"() -> ("Value"=w228:u32)  [unwired: 2 in, 2 out]
                  n158 = property on="Stop time [ms]" class="DigNum (strict)"() -> ("Value"=w226:u32)  [unwired: 2 in, 2 out]
                  n159 = property on="Current density 2 [mA/cm²]" class="DigNum (strict)"() -> ("Value"=w210:dbl)  [unwired: 2 in, 2 out]
                  n160 = property on="Current density 1 [mA/cm²]" class="DigNum (strict)"() -> ("Value"=w212:dbl)  [unwired: 2 in, 2 out]
                  n161 = Compound Arithmetic op=ADD(w230, w228, w226) -> (w234:u32)
                  n162 = Insert Into Array(array=w231, new element=w230) -> (w229:i32[])  [unwired: 1 in]
                  n163 = Add(x=w234, y=w233) -> (x+y=w232:u32)
                  n164 = Multiply(x=w212, y=w224) -> (x*y=w223:dbl)
                  n165 = Multiply(x=w224, y=w210) -> (x*y=w221:dbl)
                  n166 = Greater?(x=w232, y=w236) -> (0:w235:bool)
                  n167 = Insert Into Array(array=w229, new element=w228) -> (w227:i32[])  [unwired: 1 in]
                  n168 = Divide(x=w221, y=1000.0) -> (x/y=w216:dbl)
                  n169 = Divide(x=w223, y=1000.0) -> (x/y=w219:dbl)
                  n170 = Insert Into Array(array=w207, new element=w212) -> (w211:dbl[])  [unwired: 1 in]
                  n171 = Insert Into Array(array=w218, new element=w219) -> (w217:dbl[])  [unwired: 1 in]
                  n172 = Insert Into Array(array=w227, new element=w226) -> (w225:i32[])  [unwired: 1 in]
                  n173 = Insert Into Array(array=w217, new element=w216) -> (w215:dbl[])  [unwired: 1 in]
                  n174 = Insert Into Array(array=w211, new element=w210) -> (w209:dbl[])  [unwired: 1 in]
                  n175 = Insert Into Array(array=w215, new element=0.0 ("new element/subarray")) -> (w213:dbl[])  [unwired: 1 in]
                  n176 = Insert Into Array(array=w209, new element=0.0 ("new element/subarray")) -> (w206:dbl[])  [unwired: 1 in]
                }
                n177 = Bundle("array"=w196, "array"=w195, "array"=w194) -> (w197:T8)  [unwired: 1 in]
                n178 = Bundle By Name(cluster=w205, "Etch Program"=w197) -> (w204:T3)
              }
              frame "Non-linear Current" {
                w256 = 100 ("y")
                # "Then create arrays with increasing current"
                # "First create arrays for initial constant etch"
                # "100 ms time step"
                n179 = property on="Start Current Time [ms]" class="DigNum (strict)"() -> ("Value"=w255:u32)  [unwired: 2 in, 2 out]
                n180 = property on="Etch Surface Area [cm²]" class="DigNum (strict)"() -> ("Value"=w247:dbl)  [unwired: 2 in, 2 out]
                n181 = property on="Start Current density [mA/cm²]" class="DigNum (strict)"() -> ("Value"=w243:dbl)  [unwired: 2 in, 2 out]
                n182 = property on="Current Density Increment [mA/cm²/s^(power order)]" class="DigNum (strict)"() -> ("Value"=w239:dbl)  [unwired: 2 in, 2 out]
                n183 = Divide(x=w255, y=w256) -> (x/y=w257:dbl)
                n184 = Multiply(x=w243, y=w247) -> (x*y=w242:dbl)
                n185 = property on="Total Etch Time [s]" class="DigNum (strict)"() -> ("Value"=w253:u32)  [unwired: 2 in, 2 out]
                n186 = Round To Nearest(number=w257) -> (nearest integer value=w258:dbl)
                n187 = Divide(x=w242, y=1000.0) -> (x/y=w241:dbl)
                n188 = To Long Integer(number=w258) -> (32bit integer=w259:i32)
                n189 = Multiply(x=w253, y=1000) -> (x*y=w254:u32)
                n190 = Initialize Array(w256, w259) -> (w250:i32[])
                n191 = Initialize Array(w243, w259) -> (w249:dbl[])
                n192 = Initialize Array(w241, w259) -> (w248:dbl[])
                n193 = Subtract(x=w254, y=w255) -> (x-y=w251:u32)
                n194 = while {
                  shift-right: [w263] -> _
                  shift-left: u32 0 -> [w286]
                  tunnel: w251 -> [w285]
                  shift-right: [w281] -> w246
                  shift-left: w250 -> [w282]
                  shift-right: [w279] -> w245
                  shift-left: w249 -> [w280]
                  shift-right: [w278] -> w238
                  shift-left: w248 -> [w277]
                  tunnel: w239 -> [w275]
                  tunnel: w243 -> [w273]
                  stop <- w284 stop-if-true
                  n195 = property on="Increment time span [ms]" class="DigNum (strict)"() -> ("Value"=w283:u32)  [unwired: 2 in, 2 out]
                  n196 = property on="Increment time span [ms]" class="DigNum (strict)"() -> ("Value"=w266:u32)  [unwired: 2 in, 2 out]
                  n197 = Add(x=w283, y=w286) -> (x+y=w263:u32)
                  n198 = property on="Power order" class="DigNum (strict)"() -> ("Value"=w264:dbl)  [unwired: 2 in, 2 out]
                  n199 = To Double Precision Float(number=w263) -> (double precision float=w268:dbl)
                  n200 = property on="Etch Surface Area [cm²]" class="DigNum (strict)"() -> ("Value"=w270:dbl)  [unwired: 2 in, 2 out]
                  n201 = Greater?(x=w263, y=w285) -> (0:w284:bool)
                  n202 = Divide(x=w268, y=1000.0) -> (x/y=w265:dbl)
                  n203 = Power Of X(1:w265, 2:w264) -> (0:w276:dbl)
                  n204 = Divide(x=w270, y=1000.0) -> (x/y=w271:dbl)
                  n205 = Multiply(x=w276, y=w275) -> (x*y=w274:dbl)
                  n206 = Add(x=w274, y=w273) -> (x+y=w262:dbl)
                  n207 = Multiply(x=w262, y=w271) -> (x*y=w272:dbl)
                  n208 = Insert Into Array(array=w282, new element=w266) -> (w281:i32[])  [unwired: 1 in]
                  n209 = Insert Into Array(array=w277, new element=w272) -> (w278:dbl[])  [unwired: 1 in]
                  n210 = Insert Into Array(array=w280, new element=w262) -> (w279:dbl[])  [unwired: 1 in]
                }
                n211 = Bundle(w246, w245, w238) -> (w244:cluster{i32[], dbl[], dbl[]})  [unwired: 1 in]
                n212 = Bundle By Name(cluster=w261, "Etch Program"=w244) -> (w260:T3)
              }
            }
          }
        }
      }
      frame "Check Power Supplies" {
        # "Get Selected Power Supply Model"
        # "Checks that correct power supply is selected for the selected etch cell type. Propmts the user if power supply is incorrect."
        n213 = Unbundle By Name(w292) -> ("Etch Cell Data.Power Supply Model"=w290:string[])
        n214 = Unbundle By Name(w292) -> ("Power Supplies.Supply Model"=w295:string[])
        n215 = property on="Power Supply" class="Ring (strict)"() -> ("Value"=w294:u16)  [unwired: 2 in, 2 out]
        n216 = property on="Etch Cell" class="Slide (strict)"() -> ("Value"=w291:i32)  [unwired: 2 in, 2 out]
        n217 = Equal To 0?(x=w291) -> (x = 0?=w293:bool)
        n218 = Index Array(array=w295, index=w294) -> (element=w289:string)
        n219 = case shown="False" w293 {
          tunnel: w291 -> [w304 _]
          tunnel: w290 -> [w302 _]
          tunnel: w289 -> [w300 _]
          tunnel: [w298 w313] -> w288
          frame False {
            # "Check Power Supply model is correct for Etch\nCell selected. Case when Etch Cell Selected, not Custom Surface Area"
            n220 = Decrement(x=w304) -> (x-1=w303:i32)
            n221 = property on="Etch Cell" class="Slide (strict)" props=["Value"]() -> ()  [unwired: 2 in, 3 out]
            n222 = Index Array(array=w302, index=w303) -> (element=w301:string)
            n223 = Equal?(x=w301, y=w300) -> (x = y?=w299:bool)
            n224 = case shown="False" w299 {
              tunnel: [w307 w312] -> w298
              frame False {
                # "Power Supply model is  NOT correct for Etch\nCell selected. Ask user that it should be like that."
                n225 = Two Button Dialog(message="Selected Power Supply model does not correspond to the most suitable model for the selected Etch Cell Type.\n\nAre you sure you want to proceed with the selected Power Supply?", 1:"No, I will select another supply " ("F button name (\"Cancel\")"), 2:"Yes, Proceed" ("T button name (\"OK\")")) -> (T button?=w305:bool)
                n226 = property on="Everyting Correct" class="Bool (strict)"("Value"=w305) -> ()  [unwired: 2 in, 2 out]
                n227 = Select(t=State."Prepare Etch Program" ("Next State"), s=w305, f=State."Wait for Message") -> (s? t:f=w307:T2)
              }
              frame True {
                w312 = State."Prepare Etch Program"  # Next State
                # "Power Supply model is correct for Etch\nCell selected. Move further."
              }
            }
          }
          frame True {
            w313 = State."Prepare Etch Program"  # Next State
          }
        }
      }
      frame "Check Max Current" {
        # "Max current from etch program and lift-off pulses"
        # "Power supply Max Current from data file."
        # "Pulse 2"
        # "Pulse 1"
        # "Checks if current in the etch program and in lift-off pulses is not higher than max current for the power supply."
        n228 = Unbundle By Name(w328) -> ("Etch Program.Current [A]"=w327:dbl[])
        n229 = Unbundle By Name(w328) -> ("Power Supplies.Max Current (A)"=w330:dbl[])
        n230 = property on="Run Lift-Off Pulses\nAfter Etching" class="Bool (strict)"() -> ("Value"=w321:bool)  [unwired: 2 in, 2 out]
        n231 = property on="[A]" class="DigNum (strict)"() -> ("Value"=w323:dbl)  [unwired: 2 in, 2 out]
        n232 = property on="[A]" class="DigNum (strict)"() -> ("Value"=w322:dbl)  [unwired: 2 in, 2 out]
        n233 = Max & Min(x=w323, y=w322) -> (max(x,y)=w320:dbl)  [unwired: 1 out]
        n234 = property on="Power Supply" class="Ring (strict)"() -> ("Value"=w329:u16)  [unwired: 2 in, 2 out]
        n235 = Array Max & Min(array=w327) -> (max value=w317:dbl)  [unwired: 3 out]
        n236 = Select(t=w320, s=w321, f=0.0) -> (s? t:f=w318:dbl)
        n237 = Index Array(array=w330, index=w329) -> (element=w324:dbl)
        n238 = Max & Min(x=w317, y=w318) -> (max(x,y)=w316:dbl)  [unwired: 1 out]
        n239 = Greater Or Equal?(x=w324, y=w316) -> (x >= y?=w326:bool)
        n240 = case shown="True" w326 {
          tunnel: [w333 w343] -> w325
          tunnel: w324 -> [w341 _]
          tunnel: w316 -> [w337 _]
          frame False {
            w333 = State."Wait for Message"  # next state
            n241 = Number To Fractional String(number=w337) -> (F-format string=w336:string)  [unwired: 3 in]
            n242 = Number To Fractional String(number=w341) -> (F-format string=w340:string)  [unwired: 3 in]
            n243 = Concatenate Strings("Selected Power Supply Maximum Current is:" ("message"), w340, " A.\n\nMaximum Current during etching and/or lift-off pulses is: " ("string"), w336, " A.\n\nCheck your etch program, lift-off pulses and power supply to procced to etching." ("string")) -> (w334:string)
            n244 = One Button Dialog(message=w334, button name ("OK")="OK") -> ()  [unwired: 1 out]
            n245 = property on="Everyting Correct" class="Bool (strict)"("Value"=FALSE ("Everyting Correct")) -> ()  [unwired: 2 in, 2 out]
          }
          frame True {
            w343 = State."Prepare Graph"  # next state
          }
        }
      }
      frame "Prepare Graph" {
        w347 = T4."Enabled" ("Disabled")
        w384 = State."Wait for Message"  # next state
        # "array for current density"
        # "array for time [s]"
        n246 = Unbundle By Name(w365) -> ("Etch Program.Current Time [ms]"=w349:u32[], "Etch Program.Current Density [mA/cm2]"=w381:dbl[])
        n247 = Index Array(array=w381, index=0) -> (element=w345:dbl)
        n248 = Array Size(array=w349) -> (size(s)=w388:i32)
        n249 = Insert Into Array(array=dbl[] [], new element=w345) -> (w383:dbl[])  [unwired: 1 in]
        n250 = Insert Into Array(array=dbl[] [], new element=0.0 ("new element/subarray")) -> (w386:dbl[])  [unwired: 1 in]
        n251 = for {
          N: w388 -> [_]
          tunnel: w349 -> [w407] mode=indexing
          shift-right: [w403] -> _
          shift-left: 0 ("index") -> [w398]
          shift-right: [w406] -> w358
          shift-left: w386 -> [w396]
          tunnel: w381 -> [w392] mode=indexing
          shift-right: [w393] -> w351
          shift-left: w383 -> [w401]
          # "Buildup array with time in seconds to \ndisplay on graph"
          n252 = To Double Precision Float(number=w398) -> (double precision float=w400:dbl)
          n253 = Divide(x=w400, y=1000.0) -> (x/y=w397:dbl)
          n254 = Insert Into Array(array=w396, new element=w397) -> (w395:dbl[])  [unwired: 1 in]
          n255 = Add(x=w398, y=w407) -> (x+y=w403:u32)
          n256 = Insert Into Array(array=w401, new element=w392) -> (w394:dbl[])  [unwired: 1 in]
          n257 = To Double Precision Float(number=w403) -> (double precision float=w404:dbl)
          n258 = Divide(x=w404, y=1000.0) -> (x/y=w405:dbl)
          n259 = Insert Into Array(array=w394, new element=w392) -> (w393:dbl[])  [unwired: 1 in]
          n260 = Insert Into Array(array=w395, new element=w405) -> (w406:dbl[])  [unwired: 1 in]
        }
        n261 = property on="Start Etching" class="Bool (strict)"("DisabledEnum"=w347) -> ()  [unwired: 2 in, 2 out]
        n262 = property on="Run Lift-Off Pulses" class="Bool (strict)"("DisabledEnum"=w347) -> ()  [unwired: 2 in, 2 out]
        n263 = Array Size(array=w358) -> (size(s)=w356:i32)
        n264 = Subtract(x=w356, y=3) -> (x-y=w352:i32)
        n265 = Array Max & Min(array=w351) -> (max value=w379:dbl, min value=w378:dbl)  [unwired: 2 out]
        n266 = Initialize Array(nan, 1 ("dimension size")) -> (w361:dbl[])
        n267 = property on="Etch Surface Area [cm²]" class="DigNum (strict)"() -> ("Value"=w374:dbl)  [unwired: 2 in, 2 out]
        n268 = Array Subset(array=w358, index=0, length=w352) -> (w354:dbl[])
        n269 = Array Subset(array=w351, index=0, length=w352) -> (w350:dbl[])
        n270 = Bundle(w361, w361) -> (w359:cluster{dbl[], dbl[]})  [unwired: 1 in]
        n271 = Add(x=4.0, y=w379) -> (x+y=w372:dbl)
        n272 = Divide(x=w374, y=1000.0) -> (x/y=w368:dbl)
        n273 = Subtract(x=w378, y=4.0) -> (x-y=w369:dbl)
        n274 = Bundle(w354, w350) -> (w344:cluster{dbl[], dbl[]})  [unwired: 1 in]
        n275 = Multiply(x=w372, y=w368) -> (x*y=w371:dbl)
        n276 = Multiply(x=w369, y=w368) -> (x*y=w370:dbl)
        n277 = Bundle By Name(cluster=w365, "Graph Data"=w344) -> (w364:T3)
        n278 = Build Array(w359, w344) -> (w360:cluster{dbl[], dbl[]}[])
        n279 = property on="XY Graph" class="XYGraph (strict)"("Value"=w360, "ActYScl"=0 ("Active Y Scale"), "YScale.Maximum"=w372, "YScale.Minimum"=w369, "ActYScl"=1 ("Active Y Scale"), "YScale.Maximum"=w371, "YScale.Minimum"=w370, "XScale.Maximum"=40.0 ("X Scale.Range:Maximum"), "XScale.Minimum"=0.0 ("X Scale.Range:Minimum")) -> ()  [unwired: 2 in, 2 out]
      }
      frame "Before Etch" {
        w419 = T4."Disabled" ("Disabled")
        w424 = FALSE  # Stop Loop?
        # "Disable controls before running Etch Program"
        n280 = property on="Etch Cell" class="Slide (strict)"("DisabledEnum"=w419) -> ()  [unwired: 2 in, 2 out]
        n281 = property on="Etch Surface Area [cm²]" class="DigNum (strict)"("DisabledEnum"=w419) -> ()  [unwired: 2 in, 2 out]
        n282 = property on="Etch type" class="TabCtl (strict)"("DisabledEnum"=w419) -> ()  [unwired: 2 in, 2 out]
        n283 = property on="Pulse 1 [mA/cm²]" class="DigNum (strict)"("DisabledEnum"=w419) -> ()  [unwired: 2 in, 2 out]
        n284 = property on="Pulse 1 Time [ms]" class="DigNum (strict)"("DisabledEnum"=w419) -> ()  [unwired: 2 in, 2 out]
        n285 = property on="Pulse 2 [mA/cm²]" class="DigNum (strict)"("DisabledEnum"=w419) -> ()  [unwired: 2 in, 2 out]
        n286 = property on="Pulse 2 Time [ms]" class="DigNum (strict)"("DisabledEnum"=w419) -> ()  [unwired: 2 in, 2 out]
        n287 = property on="Wait Time [ms]" class="DigNum (strict)"("DisabledEnum"=w419) -> ()  [unwired: 2 in, 2 out]
        n288 = property on="Edit Lift-Off Pulses" class="Bool (strict)"("DisabledEnum"=w419) -> ()  [unwired: 2 in, 2 out]
        n289 = property on="Run Lift-Off Pulses\nAfter Etching" class="Bool (strict)"("DisabledEnum"=w419) -> ()  [unwired: 2 in, 2 out]
        n290 = property on="Total Etch Time [s]" class="DigNum (strict)"("DisabledEnum"=w419) -> ()  [unwired: 2 in, 2 out]
        n291 = property on="Power Supply" class="Ring (strict)"("DisabledEnum"=w419) -> ()  [unwired: 2 in, 2 out]
        n292 = property on="Everyting Correct" class="Bool (strict)"("DisabledEnum"=w419) -> ()  [unwired: 2 in, 2 out]
        n293 = property on="Exit" class="Bool"("DisabledEnum"=T4."Disabled and Grayed Out" ("Disabled")) -> ()  [unwired: 2 in, 2 out]
        n294 = Unbundle By Name(w413) -> ("Power Supplies.Max Voltage (V)"=w412:dbl[], "Power Supplies.Supply Address"=w410:string[])
        n295 = property on="Power Supply" class="Ring (strict)"() -> ("Value"=w408:u16)  [unwired: 2 in, 2 out]
        n296 = property on="Start Etching" class="Bool (strict)"() -> ("Value"=w418:bool)  [unwired: 2 in, 2 out]
        n297 = property on="Run Lift-Off Pulses" class="Bool (strict)"() -> ("Value"=w417:bool)  [unwired: 2 in, 2 out]
        n298 = Index Array(array=w412, index=w408) -> (element=w411:dbl)
        n299 = Index Array(array=w410, index=w408) -> (element=w409:string)
        n300 = Implies(1:w417, 2:w418) -> (0:w415:bool)
        n301 = Bundle By Name(cluster=w413, "Selected Voltage Limit"=w411, "Selected VISA"=w409, "Etch Finished Correctly"=FALSE, "Only LiftOff Pulses"=w415) -> (w416:T3)
        n302 = case shown="False" w415 {
          frame False {
            n303 = property on="Run Lift-Off Pulses" class="Bool (strict)"("DisabledEnum"=T4."Disabled and Grayed Out" ("Disabled")) -> ()  [unwired: 2 in, 2 out]
            n304 = property on="Start Etching" class="Bool (strict)"("BoolText.Text"="STOP\nETCH" ("Boolean Text.Text")) -> ()  [unwired: 2 in, 2 out]
          }
          frame True {
            w428 = T4."Disabled and Grayed Out" ("Disabled")
            n305 = property on="Start Etching" class="Bool (strict)"("DisabledEnum"=w428) -> ()  [unwired: 2 in, 2 out]
            n306 = property on="Run Lift-Off Pulses" class="Bool (strict)"("DisabledEnum"=w428, "BoolText.Text"="LIFT-OFF\nPULSES\nRUNNING" ("Boolean Text.Text")) -> ()  [unwired: 2 in, 2 out]
          }
        }
      }
      frame "Prepare Log" {
        w439 = FALSE  # Stop Loop?
        # "Filling Log Array"
        # "Time Etch started"
        # "Disable controls before running Etch Program"
        n307 = Unbundle By Name(w438) -> ("Only LiftOff Pulses"=w434:bool)
        n308 = Get Date/Time In Seconds() -> (seconds since 1Jan1904=w456:timestamp)
        n309 = property on="Etch Cell" class="Slide (strict)"() -> ("TextLbls[]"=w477:string[], "Value"=w476:i32)  [unwired: 2 in, 2 out]
        n310 = property on="Etch Surface Area [cm²]" class="DigNum (strict)"() -> ("Value"=w475:dbl)  [unwired: 2 in, 2 out]
        n311 = Get Date/Time String(seconds (now)=w456) -> (time string=w455:string)  [unwired: 2 in, 1 out]
        n312 = Number To Fractional String(number=w475) -> (F-format string=w474:string)  [unwired: 3 in]
        n313 = Concatenate Strings("Started: " ("string"), w455) -> (w452:string)
        n314 = Index Array(array=w477, index=w476) -> (element=w445:string)
        n315 = Initialize Array("" ("element")) -> (w451:string[])  [unwired: 1 in]
        n316 = Concatenate Strings(w445, ": " ("string"), w474, " cm2" ("string")) -> (w472:string)
        n317 = Insert Into Array(array=w451, new element=w452) -> (w450:string[])  [unwired: 1 in]
        n318 = property on="Total Etch Time [s]" class="DigNum (strict)"() -> ("Value"=w469:u32)  [unwired: 2 in, 2 out]
        n319 = Insert Into Array(array=w450, new element=w472) -> (w471:string[])  [unwired: 1 in]
        n320 = property on="Wafer Box" class="CmbBox"() -> ("Value"=w449:string)  [unwired: 2 in, 2 out]
        n321 = property on="Operator" class="CmbBox"() -> ("Value"=w431:string)  [unwired: 2 in, 2 out]
        n322 = Number To Decimal String(number=w469) -> (decimal integer string=w468:string)  [unwired: 1 in]
        n323 = Concatenate Strings("Wafer box: " ("string"), w449) -> (w448:string)
        n324 = Concatenate Strings("Operator: " ("string"), w431) -> (w429:string)
        n325 = Insert Into Array(array=w471, new element=w448) -> (w433:string[])  [unwired: 1 in]
        n326 = Concatenate Strings("Etch time: " ("string"), w468, " s" ("string")) -> (w466:string)
        n327 = case shown="False" w434 {
          tunnel: [w480 ""] -> w442
          tunnel: [w479 "Only Lift-Off Pulses Run"] -> w441
          tunnel: [State."Etch Running" ("Next State") State."LiftOff Pulses" ("Next State")] -> w437
          frame False {
            n328 = property on="Etch type" class="TabCtl (strict)"() -> ("Value"=w482:T1)  [unwired: 2 in, 2 out]
            n329 = Format Into String(format string="%s", w482) -> (resulting string=w479:string)  [unwired: 2 in, 1 out]
            n330 = case shown="\"Non-linear Current\"" w482 {
              tunnel: [w483 w487 w503] -> w480
              frame "Constant Current", Default {
                n331 = property on="Current density (mA/cm²)" class="DigNum (strict)"() -> ("Value"=w486:dbl)  [unwired: 2 in, 2 out]
                n332 = Number To Fractional String(number=w486) -> (F-format string=w485:string)  [unwired: 3 in]
                n333 = Concatenate Strings(w485, "mA/cm2" ("string")) -> (w483:string)
              }
              frame "Pulsed Etching" {
                n334 = property on="Current density 1 [mA/cm²]" class="DigNum (strict)"() -> ("Value"=w502:dbl)  [unwired: 2 in, 2 out]
                n335 = property on="Pulse time 1 [ms]" class="DigNum (strict)"() -> ("Value"=w501:u32)  [unwired: 2 in, 2 out]
                n336 = property on="Current density 2 [mA/cm²]" class="DigNum (strict)"() -> ("Value"=w500:dbl)  [unwired: 2 in, 2 out]
                n337 = property on="Pulse time 2 [ms]" class="DigNum (strict)"() -> ("Value"=w498:u32)  [unwired: 2 in, 2 out]
                n338 = property on="Stop time [ms]" class="DigNum (strict)"() -> ("Value"=w499:u32)  [unwired: 2 in, 2 out]
                n339 = Number To Fractional String(number=w502) -> (F-format string=w497:string)  [unwired: 3 in]
                n340 = Number To Decimal String(number=w501) -> (decimal integer string=w495:string)  [unwired: 1 in]
                n341 = Number To Fractional String(number=w500) -> (F-format string=w493:string)  [unwired: 3 in]
                n342 = Number To Decimal String(number=w498) -> (decimal integer string=w491:string)  [unwired: 1 in]
                n343 = Number To Decimal String(number=w499) -> (decimal integer string=w489:string)  [unwired: 1 in]
                n344 = Concatenate Strings(w497, " mA/cm2, " ("string"), w495, " ms -> " ("string"), w493, " mA/cm2, " ("string"), w491, " ms -> wait " ("string"), w489, " ms." ("string")) -> (w487:string)
              }
              frame "Non-linear Current" {
                n345 = property on="Start Current density [mA/cm²]" class="DigNum (strict)"() -> ("Value"=w514:dbl)  [unwired: 2 in, 2 out]
                n346 = property on="Start Current Time [ms]" class="DigNum (strict)"() -> ("Value"=w511:u32)  [unwired: 2 in, 2 out]
                n347 = property on="Current Density Increment [mA/cm²/s^(power order)]" class="DigNum (strict)"() -> ("Value"=w513:dbl)  [unwired: 2 in, 2 out]
                n348 = property on="Power order" class="DigNum (strict)"() -> ("Value"=w512:dbl)  [unwired: 2 in, 2 out]
                n349 = Number To Fractional String(number=w514) -> (F-format string=w510:string)  [unwired: 3 in]
                n350 = Number To Decimal String(number=w511) -> (decimal integer string=w508:string)  [unwired: 1 in]
                n351 = Number To Fractional String(number=w513) -> (F-format string=w506:string)  [unwired: 3 in]
                n352 = Number To Fractional String(number=w512) -> (F-format string=w504:string)  [unwired: 3 in]
                n353 = Concatenate Strings(w510, " mA/cm2, " ("string"), w508, " ms + " ("string"), w506, " mA/cm2 * t^" ("string"), w504) -> (w503:string)
              }
            }
          }
          frame True {
          }
        }
        n354 = Insert Into Array(array=w433, new element=w429) -> (w432:string[])  [unwired: 1 in]
        n355 = Insert Into Array(array=w432, new element=w466) -> (w465:string[])  [unwired: 1 in]
        n356 = Insert Into Array(array=w465, new element=w441) -> (w470:string[])  [unwired: 1 in]
        n357 = Insert Into Array(array=w470, new element=w442) -> (w464:string[])  [unwired: 1 in]
        n358 = property on="Run Lift-Off Pulses\nAfter Etching" class="Bool (strict)"() -> ("Value"=w435:bool)  [unwired: 2 in, 2 out]
        n359 = Or(x=w435, y=w434) -> (x .or. y?=w436:bool)
        n360 = case shown="True" w436 {
          tunnel: ["No Lift-Off pulses" w519] -> w463
          frame False {
          }
          frame True {
            n361 = property on="Pulse 2 Time [ms]" class="DigNum (strict)"() -> ("Value"=w532:u32)  [unwired: 2 in, 2 out]
            n362 = property on="Pulse 1 [mA/cm²]" class="DigNum (strict)"() -> ("Value"=w535:dbl)  [unwired: 2 in, 2 out]
            n363 = property on="Pulse 2 [mA/cm²]" class="DigNum (strict)"() -> ("Value"=w531:dbl)  [unwired: 2 in, 2 out]
            n364 = property on="Pulse 1 Time [ms]" class="DigNum (strict)"() -> ("Value"=w534:u32)  [unwired: 2 in, 2 out]
            n365 = property on="Wait Time [ms]" class="DigNum (strict)"() -> ("Value"=w533:u32)  [unwired: 2 in, 2 out]
            n366 = Number To Fractional String(number=w531) -> (F-format string=w523:string)  [unwired: 3 in]
            n367 = Number To Decimal String(number=w532) -> (decimal integer string=w521:string)  [unwired: 1 in]
            n368 = Number To Decimal String(number=w534) -> (decimal integer string=w527:string)  [unwired: 1 in]
            n369 = Number To Decimal String(number=w533) -> (decimal integer string=w525:string)  [unwired: 1 in]
            n370 = Number To Fractional String(number=w535) -> (F-format string=w529:string)  [unwired: 3 in]
            n371 = Concatenate Strings("Lift-Off: " ("string"), w529, " mA/cm2, " ("string"), w527, "ms -> wait: " ("string"), w525, " ms -> " ("string"), w523, " mA/cm2, " ("string"), w521, " ms." ("string")) -> (w519:string)
          }
        }
        n372 = Insert Into Array(array=w464, new element=w463) -> (w462:string[])  [unwired: 1 in]
        n373 = property on="Power Supply" class="Ring (strict)"() -> ("Strings []"=w460:string[], "Value"=w461:u16)  [unwired: 2 in, 2 out]
        n374 = Index Array(array=w460, index=w461) -> (element=w459:string)
        n375 = Insert Into Array(array=w462, new element=w459) -> (w457:string[])  [unwired: 1 in]
        n376 = Bundle By Name(cluster=w438, "Log"=w457) -> (w458:T3)
      }
      frame "Etch Running" {
        w566 = 0.0 ("Current Limit")
        w590 = FALSE  # Stop Loop?
        w591 = State."LiftOff Pulses"  # next state
        # "current density"
        # "time"
        # "Additional 100 ms\nso that loop does \nnot exit before \nlast array element\nfrom etch program\nis used"
        n377 = Unbundle By Name(w557) -> ("Graph Data"=w585:cluster{"X":dbl[], "Y":dbl[]})
        n378 = Unbundle By Name(w557) -> ("Selected Voltage Limit"=w555:dbl, "Selected VISA"=w556:string)
        n379 = Unbundle By Name(w557) -> ("Etch Program"=w539:T9)
        n380 = Unbundle By Name(w539) -> ("Current Time [ms]"=w542:u32[], "Current [A]"=w543:dbl[], "Current Density [mA/cm2]"=w541:dbl[])
        n381 = property on="Total Etch Time [s]" class="DigNum (strict)"() -> ("Value"=w589:u32)  [unwired: 2 in, 2 out]
        n382 = call "N5700 Initialize.vi"("VISA name"=w556, "ID Query (T)"=FALSE, "Reset (T)"=TRUE ("ID Query (T)"), "error in (no error)"=errorcluster {"status"=FALSE, "code"=0, "source"=""}) -> ("VISA out"=w563:refnum<visa-resource-name>, "error out"=w562:errorcluster)  [unwired: 10 in]
        n383 = To Double Precision Float(number=w589) -> (double precision float=w588:dbl)
        n384 = Add(x=w588, y=0.1) -> (x+y=w587:dbl)
        n385 = call "N5700 Config Voltage Limit.vi"("error"=w562, "Volt Limit"=w555, "VISA"=w563) -> ("error out"=w564:errorcluster, "VISA out"=w565:refnum<visa-resource-name>)  [unwired: 4 in]
        n386 = call "N5700 Config Output On-Off.vi"("error"=w564, "Output ON"=TRUE, "VISA"=w565) -> ("error out"=w559:errorcluster, "VISA out"=w560:refnum<visa-resource-name>)  [unwired: 4 in]
        n387 = Array Size(array=w541) -> (size(s)=w540:i32)
        n388 = for {
          N: w540 -> [_]
          tunnel: w587 -> [w646]
          tunnel: w585 -> [w642]
          tunnel: w560 -> [w632]
          tunnel: w559 -> [w631]
          tunnel: [w626] -> w581
          tunnel: [w625] -> w580
          tunnel: [w623] -> w577
          tunnel: [w622] -> w549
          tunnel: [w598] -> w575
          tunnel: [w623] -> w573
          tunnel: [w596] -> w551
          shift-right: [w613] -> _
          shift-left: dbl[] [] ("X") -> [w618]
          shift-right: [w614] -> _
          shift-left: dbl[] [] ("Y") -> [w616]
          shift-right: [w606] -> w544
          shift-left: w545 -> [w607]
          tunnel: w541 -> [w605] mode=indexing
          tunnel: w543 -> [w604] mode=indexing
          tunnel: w542 -> [w603] mode=indexing
          shift-right: [w601] -> w536
          shift-left: w538 -> [w602]
          i -> [w596]
          stop <- w624 stop-if-true
          w636 = 20.0 ("x")
          # "This part rescale graph X axis\nduring etching time"
          n389 = Equal To 0?(x=w596) -> (x = 0?=w645:bool)
          n390 = Dequeue Element(queue=w607, timeout in ms (-1)=5, error in (no error)=w602) -> (queue out=w606:refnum<queue>, element=w600:T2, error out=w601:errorcluster)  [unwired: 1 out]
          n391 = To Double Precision Float(number=w603) -> (double precision float=w610:dbl)
          n392 = call "Elapsed Time"("Time Target (s)"=w646, "Reset"=w645) -> ("Elapsed Time (s)"=w612:dbl, "Time has Elapsed"=w622:bool)  [unwired: 10 in, 6 out]
          n393 = Divide(x=w610, y=1000.0) -> (x/y=w609:dbl)
          n394 = Insert Into Array(array=w616, new element=w612) -> (w615:dbl[])  [unwired: 1 in]
          n395 = Insert Into Array(array=w618, new element=w605) -> (w617:dbl[])  [unwired: 1 in]
          n396 = call "N5700 Config Current Limit.vi"("error"=w631, "Current Limit"=w604, "VISA"=w632) -> ("error out"=w629:errorcluster, "VISA out"=w630:refnum<visa-resource-name>)  [unwired: 4 in]
          n397 = property on="Current now [A]" class="DigNum (strict)"("Value"=w604) -> ()  [unwired: 2 in, 2 out]
          n398 = Add(x=w612, y=w609) -> (x+y=w611:dbl)
          n399 = Equal?(x=w600, y=State."Stop Etch Clicked") -> (x = y?=w598:bool)
          n400 = Insert Into Array(array=w617, new element=w605) -> (w613:dbl[])  [unwired: 1 in]
          n401 = Insert Into Array(array=w615, new element=w611) -> (w614:dbl[])  [unwired: 1 in]
          n402 = call "N5700 Wait.vi"("error"=w629, "Delay (5 mS)"=w603, "VISA"=w630) -> ("error out"=w628:errorcluster, "VISA out"=w627:refnum<visa-resource-name>)  [unwired: 4 in]
          n403 = Add(x=w636, y=w612) -> (x+y=w641:dbl)
          n404 = Multiply(x=w604, y=0.5) -> (x*y=w620:dbl)
          n405 = property on="Elapsed Time [s]" class="DigNum (strict)"("Value"=w612) -> ()  [unwired: 2 in, 2 out]
          n406 = call "N5700 Meas Output Current.vi"("error"=w628, "VISA"=w627) -> ("error out"=w625:errorcluster, "Output Current"=w619:dbl, "VISA out"=w626:refnum<visa-resource-name>)  [unwired: 4 in]
          n407 = Multiply(x=w636, y=2.0) -> (x*y=w639:dbl)
          n408 = Bundle("Y"=w614, "X"=w613) -> (w643:cluster{"Y":dbl[], "X":dbl[]})  [unwired: 1 in]
          n409 = Subtract(x=w612, y=w636) -> (x-y=w635:dbl)
          n410 = Greater Or Equal?(x=w612, y=w636) -> (x >= y?=w637:bool)
          n411 = Less?(x=w619, y=w620) -> (x < y?=w623:bool)
          n412 = Select(t=w641, s=w637, f=w639) -> (s? t:f=w640:dbl)
          n413 = Select(t=w635, s=w637, f=0.0) -> (s? t:f=w633:dbl)
          n414 = Build Array(w643, w642) -> (w644:cluster{"X":dbl[], "Y":dbl[]}[])
          n415 = Quotient & Remainder(x=w596, y=3) -> (floor(x/y)=w597:i32)  [unwired: 1 out]
          n416 = property on="XY Graph" class="XYGraph (strict)"("Value"=w644, "XScale.Maximum"=w640, "XScale.Minimum"=w633) -> ()  [unwired: 2 in, 2 out]
          n417 = property on="Number of layers" class="DigNum (strict)"("Value"=w597) -> ()  [unwired: 2 in, 2 out]
          n418 = Compound Arithmetic op=OR(w623, w598, w622) -> (w624:bool)
        }
        n419 = Decrement(x=w540) -> (x-1=w552:i32)
        n420 = Equal?(x=w551, y=w552) -> (x = y?=w550:bool)
        n421 = case shown="True" w577 {
          frame False {
          }
          frame True {
            n422 = One Button Dialog(message="Power Supply did not give current. Check the connectors to etching cell and connection to Pt wires. Then try again. ", button name ("OK")="OK") -> ()  [unwired: 1 out]
          }
        }
        n423 = Or(x=w549, y=w550) -> (x .or. y?=w548:bool)
        n424 = call "N5700 Config Current Limit.vi"("error"=w580, "Current Limit"=w566, "VISA"=w581) -> ("error out"=w583:errorcluster, "VISA out"=w584:refnum<visa-resource-name>)  [unwired: 4 in]
        n425 = property on="Current now [A]" class="DigNum (strict)"("Value"=w566) -> ()  [unwired: 2 in, 2 out]
        n426 = Select(t="No current" ("button name (\"OK\")"), s=w573, f="") -> (s? t:f=w569:string)
        n427 = Select(t="Aborted by user" ("button name (\"OK\")"), s=w575, f="") -> (s? t:f=w570:string)
        n428 = Concatenate Strings(w569, w570) -> (w571:string)
        n429 = Bundle By Name(cluster=w557, "Etch Result"=w571, "Etch Finished Correctly"=w548) -> (w576:T3)
        n430 = call "N5700 Config Output On-Off.vi"("error"=w583, "Output ON"=FALSE, "VISA"=w584) -> ("error out"=w579:errorcluster, "VISA out"=w578:refnum<visa-resource-name>)  [unwired: 4 in]
        n431 = call "N5700 Close.vi"("error"=w579, "VISA name"=w578) -> ()  [unwired: 6 in, 1 out]
        n432 = Merge Errors(w536, w538) -> (w537:errorcluster)
      }
      frame "LiftOff Pulses" {
        n433 = flat-sequence {
          tunnel: w650 -> [w661]
          tunnel: w649 -> [w660]
          tunnel: w648 -> [w659]
          frame #0 {
            n434 = Unbundle By Name(w659) -> ("Etch Finished Correctly"=w657:bool, "Only LiftOff Pulses"=w654:bool)
            n435 = property on="Run Lift-Off Pulses\nAfter Etching" class="Bool (strict)"() -> ("Value"=w658:bool)  [unwired: 2 in, 2 out]
            n436 = And(x=w658, y=w657) -> (x .and. y?=w656:bool)
            n437 = Or(x=w656, y=w654) -> (x .or. y?=w655:bool)
            n438 = case shown="True" w655 {
              tunnel: w661 -> [_ w691]
              tunnel: w660 -> [_ w690]
              frame False {
              }
              frame True {
                n439 = call "N5700 Initialize.vi"("VISA name"=w691, "ID Query (T)"=FALSE, "Reset (T)"=TRUE ("ID Query (T)"), "error in (no error)"=errorcluster {"status"=FALSE, "code"=0, "source"=""}) -> ("VISA out"=w695:refnum<visa-resource-name>, "error out"=w694:errorcluster)  [unwired: 10 in]
                n440 = call "N5700 Config Voltage Limit.vi"("error"=w694, "Volt Limit"=w690, "VISA"=w695) -> ("error out"=w696:errorcluster, "VISA out"=w697:refnum<visa-resource-name>)  [unwired: 4 in]
                n441 = call "N5700 Config Output On-Off.vi"("error"=w696, "Output ON"=TRUE, "VISA"=w697) -> ("error out"=w689:errorcluster, "VISA out"=w688:refnum<visa-resource-name>)  [unwired: 4 in]
                n442 = property on="[A]" class="DigNum (strict)"() -> ("Value"=w687:dbl)  [unwired: 2 in, 2 out]
                n443 = property on="Pulse 1 Time [ms]" class="DigNum (strict)"() -> ("Value"=w684:u32)  [unwired: 2 in, 2 out]
                n444 = call "N5700 Config Current Limit.vi"("error"=w689, "Current Limit"=w687, "VISA"=w688) -> ("error out"=w685:errorcluster, "VISA out"=w686:refnum<visa-resource-name>)  [unwired: 4 in]
                n445 = call "N5700 Wait.vi"("error"=w685, "Delay (5 mS)"=w684, "VISA"=w686) -> ("error out"=w670:errorcluster, "VISA out"=w672:refnum<visa-resource-name>)  [unwired: 4 in]
                n446 = property on="Wait Time [ms]" class="DigNum (strict)"() -> ("Value"=w677:u32)  [unwired: 2 in, 2 out]
                n447 = call "N5700 Config Current Limit.vi"("error"=w670, "Current Limit"=0.0, "VISA"=w672) -> ("error out"=w669:errorcluster, "VISA out"=w671:refnum<visa-resource-name>)  [unwired: 4 in]
                n448 = call "N5700 Wait.vi"("error"=w669, "Delay (5 mS)"=w677, "VISA"=w671) -> ("error out"=w678:errorcluster, "VISA out"=w679:refnum<visa-resource-name>)  [unwired: 4 in]
                n449 = property on="[A]" class="DigNum (strict)"() -> ("Value"=w681:dbl)  [unwired: 2 in, 2 out]
                n450 = property on="Pulse 2 Time [ms]" class="DigNum (strict)"() -> ("Value"=w680:u32)  [unwired: 2 in, 2 out]
                n451 = call "N5700 Config Current Limit.vi"("error"=w678, "Current Limit"=w681, "VISA"=w679) -> ("error out"=w683:errorcluster, "VISA out"=w682:refnum<visa-resource-name>)  [unwired: 4 in]
                n452 = call "N5700 Wait.vi"("error"=w683, "Delay (5 mS)"=w680, "VISA"=w682) -> ("error out"=w675:errorcluster, "VISA out"=w676:refnum<visa-resource-name>)  [unwired: 4 in]
                n453 = call "N5700 Config Current Limit.vi"("error"=w675, "Current Limit"=0.0, "VISA"=w676) -> ("error out"=w667:errorcluster, "VISA out"=w668:refnum<visa-resource-name>)  [unwired: 4 in]
                n454 = call "N5700 Config Output On-Off.vi"("error"=w667, "Output ON"=FALSE, "VISA"=w668) -> ("error out"=w663:errorcluster, "VISA out"=w664:refnum<visa-resource-name>)  [unwired: 4 in]
                n455 = call "N5700 Close.vi"("error"=w663, "VISA name"=w664) -> ()  [unwired: 6 in, 1 out]
              }
            }
          }
          frame #1 {
            n456 = call <vilib>:"Application Directory.vi"() -> ("Application Directory"=w702:path)
            n457 = Build Path(base path=w702, name or relative path="sounds") -> (appended path=w700:path)
            n458 = Build Path(base path=w700, name or relative path="EtchEnd.wav") -> (appended path=w698:path)
            n459 = call <vilib>:"Play Sound File.vi"("path"=w698) -> ()  [unwired: 9 in, 2 out]
          }
        }
        n460 = Unbundle By Name(w648) -> ("Selected Voltage Limit"=w649:dbl, "Selected VISA"=w650:string)
      }
      frame "After Etch" {
        w706 = FALSE  # Stop Loop?
        w703 = State."Wait for Message"  # next state
        n461 = flat-sequence {
          tunnel: w705 -> [w716]
          frame #0 {
            n462 = Unbundle By Name(w716) -> ("Log"=w715:string[], "Etch Finished Correctly"=w710:bool, "Only LiftOff Pulses"=w708:bool, "Etch Result"=w709:string)
            n463 = Array Size(array=w715) -> (size(s)=w714:i32)
            n464 = Or(x=w710, y=w708) -> (x .or. y?=w711:bool)
            n465 = Greater?(x=w714, y=1) -> (0:w712:bool)
            n466 = case shown="True" w712 {
              tunnel: w711 -> [_ w734]
              tunnel: w709 -> [_ w733]
              tunnel: w715 -> [_ w717]
              frame False {
              }
              frame True {
                n467 = Get Date/Time In Seconds() -> (seconds since 1Jan1904=w724:timestamp)
                n468 = Select(t="Finished correctly", s=w734, f=w733) -> (s? t:f=w720:string)
                n469 = call <vilib>:"Application Directory.vi"() -> ("Application Directory"=w729:path)
                n470 = Format Date/Time String(time format string (%c)="%Y_%m_%d", seconds (now)=w724) -> (date/time string=w722:string)  [unwired: 1 in]
                n471 = Build Path(base path=w729, name or relative path="logs") -> (appended path=w727:path)
                n472 = Concatenate Strings("Result: " ("string"), w720) -> (w718:string)
                n473 = Insert Into Array(array=w717, new element=w718) -> (w731:string[])  [unwired: 1 in]
                n474 = Concatenate Strings(w722, ".csv" ("string")) -> (w725:string)
                n475 = Build Path(base path=w727, name or relative path=w725) -> (appended path=w721:path)
                n476 = call-poly <vilib>:"Write Delimited Spreadsheet.vi"("file path (dialog if empty)"=w721, "1D data"=w731, "append to file? (new file:F)"=TRUE) -> ()  [unwired: 11 in, 2 out]
              }
            }
          }
          frame #1 {
            w737 = T4."Disabled and Grayed Out" ("Disabled")
            w735 = T4."Enabled" ("Disabled")
            n477 = property on="Everyting Correct" class="Bool (strict)"("Value"=FALSE ("Everyting Correct")) -> ()  [unwired: 2 in, 2 out]
            n478 = property on="Etch Cell" class="Slide (strict)"("DisabledEnum"=w735) -> ()  [unwired: 2 in, 2 out]
            n479 = property on="Etch Surface Area [cm²]" class="DigNum (strict)"("DisabledEnum"=w735) -> ()  [unwired: 2 in, 2 out]
            n480 = property on="Etch type" class="TabCtl (strict)"("DisabledEnum"=w735) -> ()  [unwired: 2 in, 2 out]
            n481 = property on="Pulse 1 Time [ms]" class="DigNum (strict)"("DisabledEnum"=w735) -> ()  [unwired: 2 in, 2 out]
            n482 = property on="Pulse 1 [mA/cm²]" class="DigNum (strict)"("DisabledEnum"=w735) -> ()  [unwired: 2 in, 2 out]
            n483 = property on="Pulse 2 Time [ms]" class="DigNum (strict)"("DisabledEnum"=w735) -> ()  [unwired: 2 in, 2 out]
            n484 = property on="Pulse 2 [mA/cm²]" class="DigNum (strict)"("DisabledEnum"=w735) -> ()  [unwired: 2 in, 2 out]
            n485 = property on="Wait Time [ms]" class="DigNum (strict)"("DisabledEnum"=w735) -> ()  [unwired: 2 in, 2 out]
            n486 = property on="Edit Lift-Off Pulses" class="Bool (strict)"("DisabledEnum"=w735) -> ()  [unwired: 2 in, 2 out]
            n487 = property on="Run Lift-Off Pulses\nAfter Etching" class="Bool (strict)"("DisabledEnum"=w735) -> ()  [unwired: 2 in, 2 out]
            n488 = property on="Total Etch Time [s]" class="DigNum (strict)"("DisabledEnum"=w735) -> ()  [unwired: 2 in, 2 out]
            n489 = property on="Everyting Correct" class="Bool (strict)"("DisabledEnum"=w735) -> ()  [unwired: 2 in, 2 out]
            n490 = property on="Power Supply" class="Ring (strict)"("DisabledEnum"=w735) -> ()  [unwired: 2 in, 2 out]
            n491 = property on="Exit" class="Bool"("DisabledEnum"=w735) -> ()  [unwired: 2 in, 2 out]
            n492 = property on="Start Etching" class="Bool (strict)"("Value"=FALSE ("Start Etching"), "BoolText.Text"="START\nETCH" ("Boolean Text.Text"), "DisabledEnum"=w737) -> ()  [unwired: 2 in, 2 out]
            n493 = property on="Run Lift-Off Pulses" class="Bool (strict)"("Value"=FALSE ("Run Lift-Off Pulses"), "DisabledEnum"=w737, "BoolText.Text"="RUN\nLIFT-OFF\nPULSES" ("Boolean Text.Text")) -> ()  [unwired: 2 in, 2 out]
          }
        }
      }
      frame "Exit" {
        w744 = TRUE  # Stop Loop?
        w746 = State."Exit"  # (Value Not Used)
        # "#CodeNeeded - Add any required cleanup code here."
        # "The state value is not used here since this is the last iteration of the state machine loop."
        # "Exit - Exit the application."
      }
      frame "Stop Etch Clicked" {
        # "This case should be never reached. This is dummy case for the Etch Running case to indicate that etching loop must be stopped."
      }
    }
    n494 = Or(x=w15, y=w17) -> (x .or. y?=w16:bool)
  }
  n495 = while {
    shift-right: [w756] -> w6
    shift-left: w3 -> [w757]
    shift-right: [w754] -> _
    shift-left: w7 -> [w755]
    stop <- w753 stop-if-true
    # "User Event Handling Loop"
    n496 = event shown="[5] \"Current density (mA/cm²)\", \"Current density 1 [mA/cm²]\", \"Current density 2 [mA/cm²]\", \"Pulse time 1 [ms]\", \"Pulse time 2 [ms]\", \"Stop time [ms]\", \"Start Current Time [ms]\", \"Start Current density [mA/cm²]\", \"Power order\", \"Increment time span [ms]\", \"Current Density Increment [mA/cm²/s^(power order)]\", \"Total Etch Time [s]\", \"Wafer Box\", \"Run Lift-Off Pulses After Etching\", \"Pulse 1 Time [ms]\", \"Pulse 2 Time [ms]\", \"Wait Time [ms]\": Value Change" {
      selector: _ -> [_ _ _ _ _ _ _ _ _ _]
      dyn-events: _ -> [_ _ _ _ _ _ _ _ _ _]
      timeout: _ -> [_ _ _ _ _ _ _ _ _ _]
      tunnel: w757 -> [w762 w767 w772 w777 w782 w787 w792 w807 w811 w814]
      tunnel: [w760 w766 w771 w776 w781 w786 w791 w806 w812 w817] -> w756
      tunnel: w755 -> [w759 w765 w770 w775 w780 w784 w790 w805 w810 w816]
      tunnel: [w758 w764 w769 w774 w779 w785 w789 w804 w809 w815] -> w754
      tunnel: [_ _ _ _ _ _ _ _ _ TRUE] -> w752
      event "Etch Cell": Value Change {
        n497 = event-data() -> ()  [unwired: 1 in, 1 out]
        n498 = Enqueue Element(queue=w762, element=State."Etch Cell Changed", error in (no error)=w759) -> (queue out=w760:refnum<queue>, error out=w758:errorcluster)  [unwired: 1 in, 1 out]
      }
      event "Pulse 1 [mA/cm²]", "Pulse 2 [mA/cm²]": Value Change {
        n499 = event-data() -> ()  [unwired: 1 in, 1 out]
        n500 = Enqueue Element(queue=w767, element=State."LiftOff Pulse Changed", error in (no error)=w765) -> (queue out=w766:refnum<queue>, error out=w764:errorcluster)  [unwired: 1 in, 1 out]
      }
      event "Edit Lift-Off Pulses": Value Change {
        n501 = event-data() -> ()  [unwired: 1 in, 1 out]
        n502 = Enqueue Element(queue=w772, element=State."Enable Editing Pulses Clicked", error in (no error)=w770) -> (queue out=w771:refnum<queue>, error out=w769:errorcluster)  [unwired: 1 in, 1 out]
      }
      event "Etch type": Value Change {
        n503 = event-data() -> ()  [unwired: 1 in, 1 out]
        n504 = Enqueue Element(queue=w777, element=State."Etch Type Changed", error in (no error)=w775) -> (queue out=w776:refnum<queue>, error out=w774:errorcluster)  [unwired: 1 in, 1 out]
      }
      event "Refresh Supplies": Value Change {
        n505 = event-data() -> ()  [unwired: 1 in, 1 out]
        n506 = Enqueue Element(queue=w782, element=State."Refresh Supplies Clicked", error in (no error)=w780) -> (queue out=w781:refnum<queue>, error out=w779:errorcluster)  [unwired: 1 in, 1 out]
      }
      event "Current density (mA/cm²)", "Current density 1 [mA/cm²]", "Current density 2 [mA/cm²]", "Pulse time 1 [ms]", "Pulse time 2 [ms]", "Stop time [ms]", "Start Current Time [ms]", "Start Current density [mA/cm²]", "Power order", "Increment time span [ms]", "Current Density Increment [mA/cm²/s^(power order)]", "Total Etch Time [s]", "Wafer Box", "Run Lift-Off Pulses\nAfter Etching", "Pulse 1 Time [ms]", "Pulse 2 Time [ms]", "Wait Time [ms]": Value Change {
        n507 = event-data() -> ()  [unwired: 1 in, 1 out]
        n508 = Enqueue Element(queue=w787, element=State."Etch Parameters Changed", error in (no error)=w784) -> (queue out=w786:refnum<queue>, error out=w785:errorcluster)  [unwired: 1 in, 1 out]
      }
      event "Start Etching": Value Change {
        n509 = event-data() -> ()  [unwired: 1 in, 1 out]
        n510 = property on="Start Etching" class="Bool (strict)"() -> ("Value"=w788:bool)  [unwired: 2 in, 2 out]
        n511 = case shown="False" w788 {
          tunnel: w792 -> [w797 w802]
          tunnel: [w796 w801] -> w791
          tunnel: w790 -> [w795 w800]
          tunnel: [w794 w799] -> w789
          frame False {
            n512 = Enqueue Element(queue=w797, element=State."Stop Etch Clicked", error in (no error)=w795) -> (queue out=w796:refnum<queue>, error out=w794:errorcluster)  [unwired: 1 in, 1 out]
          }
          frame True {
            n513 = Enqueue Element(queue=w802, element=State."Before Etch", error in (no error)=w800) -> (queue out=w801:refnum<queue>, error out=w799:errorcluster)  [unwired: 1 in, 1 out]
          }
        }
      }
      event "Run Lift-Off Pulses": Value Change {
        n514 = event-data() -> ()  [unwired: 1 in, 1 out]
        n515 = Enqueue Element(queue=w807, element=State."Before Etch", error in (no error)=w805) -> (queue out=w806:refnum<queue>, error out=w804:errorcluster)  [unwired: 1 in, 1 out]
      }
      event "Everyting Correct": Value Change {
        n516 = event-data() -> ()  [unwired: 1 in, 1 out]
        n517 = Enqueue Element(queue=w811, element=State."Prepare Etch Program", error in (no error)=w810) -> (queue out=w812:refnum<queue>, error out=w809:errorcluster)  [unwired: 1 in, 1 out]
      }
      event "Exit": Value Change {
        n518 = event-data() -> ()  [unwired: 1 in, 1 out]
        n519 = Enqueue Element(queue=w814, element=State."Exit", error in (no error)=w816) -> (queue out=w817:refnum<queue>, error out=w815:errorcluster)  [unwired: 1 in, 1 out]
      }
    }
    n520 = Or(x=w754, y=w752) -> (x .or. y?=w753:bool)
  }
  n521 = Release Queue(queue=w6, error in (no error)=w2) -> (error out=w1:errorcluster)  [unwired: 1 in, 2 out]
  n522 = call <vilib>:"Simple Error Handler.vi"("error in (no error)"=w1) -> ("error out"=w8:errorcluster)  [unwired: 4 in, 4 out]
  n523 = disable-structure shown="RUN_TIME_ENGINE==True" {
    disable-tunnel: w8 -> [_ _]
    frame condition #0 (active) {
    }
    frame condition #1 {
      # "Call Quit LabVIEW if running as a built application."
      n524 = Quit LabVIEW() -> ()  [unwired: 1 in]
    }
  }
